vi "Check LVDT's Position.vi"(6 "lvdt display in":T1[](array[typedef]) {"value" format="%.2f"}, 8 "System Error In":errorcluster, 9 "check lvdt x?":bool, 10 "input cluster":T2={"Application Status"="", "Switch Output Array"=[], "Switch Value Configuration"=[], "NVH Configuration"={"NVH Station?"=FALSE, "nvh app instance path"="", "NVH_ErrorMessages sv url"="", "NVH_Inputs sv url"="", "NVH_MotionNumber sv url"="", "NVH_Outputs sv url"="", "NVH_PartNumber sv url"="", "NVH_PartNumber_Echo sv url"="", "NVH_SerialNumber sv url"="", "NVH_AmbientTempF sv url"=""}, "rs232 port map"={"PMAC"="", "PS Port"="", "LVDT Unit"="", "RS232"=""}, "ethernet address map"={"LVDT 1 Unit"="172.17.53.143", "LVDT Unit 1 port"=0}, "paths"={"Base Path"=path "", "system error log path"=path "", "Error Table Path"=path "C/Labview Code/System/Error Table", "Store errors log path"=path "C/Labview Code/System/Error Table", "data bytes log path"=path "C/Labview Code/System/Error Table", "network path"=path "C/Labview Code/System/Error Table"}, "Station Index"=0, "Store Data"={"Motion Data Array"=[], "Error Table"=[], "Sun Shade Close Force Limits"={"Overall Min"=0.0, "Overall Max"=0.0, "Avg Min"=0.0, "Avg Max"=0.0, "Truncation Start"=0.0, "Truncation End"=0.0, "Variance"=0.0, "Check Noise"=FALSE}, "Sun Shade Open Force Limits"={"Overall Min"=0.0, "Overall Max"=0.0, "Avg Min"=0.0, "Avg Max"=0.0, "Truncation Start"=0.0, "Truncation End"=0.0, "Variance"=0.0, "Check Noise"=FALSE}, "Sunshade Open Data"=[], "Sunshade Close Data"=[], "Module Info"={"Serial Number"="", "Pallet Number"="", "Sunshade Color"="", "Inalfa Part Number"="", "Customer Number"=""}, "Sunsahde Close Raw Data"=[], "Sunshade Open Raw Data"=[], "Software Version"=[], "Constant Version"=[], "Hardware Version"=[], "Inalfa Part Number ECU"=[], "LVDT Data"=[], "Communication Line 1"=[], "Communication Line 2"=[], "Anti Pinch Force"=[], "Cycle Time"="", "Anti Pinch Vent Force"=[], "iGPS LVDT Data"=[], "data bytes log"=""}, "D in map"={"Abort Test"=enum."Dev2/port2/line6", "Start Test"=enum."Dev2/port2/line6"}, "DO Task"="", "ctl refs"={"Start Test"=refnum, "Abort Test"=refnum, "Manual Control"=refnum, "Route to Repair"=refnum, "Waveform Graph"=refnum, "Motion Data"=refnum, "all station status"=refnum, "Individual Station Status"=refnum, "exit program"=refnum, "Sunshade Servo Data Open"=refnum, "Sunshade Servo Data Close"=refnum, "Red-Rabbit Mode"=refnum, "Direct Manual Ctrl"=refnum}, "misc station config"={"Station Name"="", "is AT station?"=FALSE, "is audit station?"=FALSE, "power supply type"=enum."GENser", "use alt China TP2 LVDT Logic Seq"=FALSE, "hmi operator abort timeout"=0, "dump all analog values even if pass"=FALSE, "debug log pre-filter ap stream bytes"=FALSE, "use separate lvdt x and z extend tags"=FALSE, "is print"=FALSE}, "ethernet tcp refs"={"LVDT Unit"=refnum}, "Sunshade Barcode Scan"={"Sunshade Number 2"="", "Sunshade Number 1"="", "Keyence tuning bank idx"=0}, "AP Test Data"={"Raw Sunshade AP Data"="", "Raw Glass AP Data"="", "PMAC Read Counter"=0.0, "Database AP Data"=[]}, "Motion Status"={"hmi operator abort start time"=0, "Current Data Index"=0, "Analog Data"=[], "Motor Position Hex"=0, "Messages Index"=0, "Last Bytes"=[], "Current Hall Position"=0, "Motion Stop Timer"=0, "Position Test"=enum."Not Tested", "Noise Test"=enum."Not Tested", "motion stop check initialized"=FALSE, "remote sense enabled"=FALSE, "Motion"=enum."Glass Teach"}, "LVDT Status"={"LVDT's stored config"=[], "lvdt precision"={"truncate instead of rounding"=FALSE, "decimal places"=0}}, "Sequence State"={"Step Description"="", "Cycle Start Time"=0, "Step Data String"="", "Pass?"=FALSE, "Seqence"=[], "Active Step"=0, "Testing?"=FALSE, "Red-Rabbit Mode"=FALSE, "route-to-repair mode"=FALSE, "NVH Status"={"Restart IRQ Counter"=0, "NVH Test Needed?"=FALSE, "NVH Test Running?"=FALSE}, "Present (s)"=0.0, "Hold Mode?"=FALSE, "Hold?"=FALSE, "Rx Invalid?"=FALSE}, "misc status"={"delay start time (ticks)"=0, "In Vehicle Mode?"=FALSE, "Diag Mode?"=FALSE, "Serial Port Configured?"=FALSE, "PS Voltage"=0.0, "Diag Serial Port"="", "Part Setup"={"Communication Type"=enum."None", "Send Messages to"=enum."Glass", "RAP Signal"=enum."High", "Motor Type"=enum."Smart Motor", "NVH Part Number"=0, "Turn Off Timer"=0, "Part Type"=""}, "Part History Number"="", "Plant Number"=0, "AP Data Type"=enum."91/61", "Real Rollo?"=FALSE}, "NVH Operator?"=FALSE, "NVH Pass?"=FALSE, "Operator Pass?"=FALSE, "Operator Action?"=FALSE, "Noise Source"=0, "USBHandle"=0, "PeakInfo"="", "PeakNumber"=0, "NVH Motion Steps"=[], "Second Check?"=FALSE, "Decibel data"=[], "Direct Control Info"={"EnableStopOnHome"=FALSE, "EnableStopOnPos"=FALSE, "TeachEvent"=FALSE, "open offset"=0, "close offset"=0, "Derect control"=FALSE, "set position"=[], "teach pass "=FALSE, "Drift offsets"=[], "Hall Positions"=[]}, "manual control(direct)"=FALSE, "LIN INFO"={"Toolkit Type"=enum."Inalfa LIN", "NAD"=36, "Inalfa LIN"={"Master Frame(3C)"="", "Slave Frame(3D)"="NIXNET_exampleLDF", "Request Schedule"="NIXNET_exampleLDF", "Response Schedule"="CEMLIN3DiagResponseSchedule\nSPA3414_ConfigurationsCMAGeely_CEMCALYPSOSDB34XX0Cfg_LIN3_190709_", "Frame Write SCU"="", "Frame Read SCU"="", "LIN Name"=""}, "ADCS LIN"={"Port"="MasterReq\nSPA3414_ConfigurationsCMAGeely_CEMCALYPSOSDB34XX0Cfg_LIN3_190709_", "HW select"=0, "XNET Cluster"="SlaveResp\nSPA3414_ConfigurationsCMAGeely_CEMCALYPSOSDB34XX0Cfg_LIN3_190709_", "ByteCmd Path"=path "C/Labview Code/System/ByteCmdConfig.txt"}, "TS LIN"={"ref info"=refnum, "LIN Channel"=0, "ByteCmd Path"=path "C/Labview Code/System/ByteCmdConfig.txt"}}, "Config Info"=variant} {"LIN INFO"."NAD" format="%.0x"; "LIN INFO"."ADCS LIN"."HW select" items=["NI-XNET", "NI-CAN"]; "LVDT Status"."LVDT's stored config"."Lower Limit" format="%.2f"; "LVDT Status"."LVDT's stored config"."Upper Limit" format="%.2f"; "Store Data"."Sun Shade Open Force Limits"."Variance" format="%.2g"; "Store Data"."Sun Shade Open Force Limits"."Truncation End" format="%.2g"; "Store Data"."Sun Shade Open Force Limits"."Truncation Start" format="%.2g"; "Store Data"."Sun Shade Open Force Limits"."Avg Max" format="%.2g"; "Store Data"."Sun Shade Open Force Limits"."Avg Min" format="%.2g"; "Store Data"."Sun Shade Open Force Limits"."Overall Max" format="%.2g"; "Store Data"."Sun Shade Open Force Limits"."Overall Min" format="%.2g"; "Store Data"."Sun Shade Close Force Limits"."Variance" format="%.2g"; "Store Data"."Sun Shade Close Force Limits"."Truncation End" format="%.2g"; "Store Data"."Sun Shade Close Force Limits"."Truncation Start" format="%.2g"; "Store Data"."Sun Shade Close Force Limits"."Avg Max" format="%.2g"; "Store Data"."Sun Shade Close Force Limits"."Avg Min" format="%.2g"; "Store Data"."Sun Shade Close Force Limits"."Overall Max" format="%.2g"; "Store Data"."Sun Shade Close Force Limits"."Overall Min" format="%.2g"}, 11 "Database LVDT's Data In":sgl[](array[numeric])) -> (0 "System Error Out":errorcluster, 1 "Error String Number":u16[](array[numeric]), 2 "Error String Array":string[](array[string]), 3 "Database LVDT's Data Out":sgl[](array[numeric]), 4 "lvdt display out":T1[](array[typedef]) {"value" format="%.2f"}, 5 "Pass?":bool)   [LabVIEW 2018]
uses:
  type defs/EOL LVDT's Check Controller.ctl
  02.Type Def's/lvdt name val pair.ctl
  <vilib>/Platform/dataskt.llb/DataSocket Reference Type.ctl
  type defs/plc path and tag.ctl
  02.Type Def's/station plc write boolean tags.ctl
  02.Type Def's/station plc read boolean tags.ctl
  type defs/EOL Global Digital Input Control.ctl
  02.Type Def's/station DI map.ctl
  lvdt precision.ctl
  02.Type Def's/All Communication Types.ctl
  type defs/Communication with Motors.ctl
  type defs/RAP Signal Control.ctl
  type defs/EOL Motor Type.ctl
  type defs/EOL Part Setup.ctl
  type defs/17x AP Data Type.ctl
  02.Type Def's/All Motions.ctl
  02.Type Def's/EOL Switch Max Min Check Cluster.ctl
  02.Type Def's/EOL Switch Value Configuration Cluster.ctl
  02.Type Def's/All Switch Configuration Cluster.ctl
  type defs/17x Sunshade Limts Seq.ctl
  02.Type Def's/Pass Fail Control.ctl
  02.Type Def's/EOL Module Info Control.ctl
  type defs/17x Audit Motion Data Seq Control.ctl
  02.Type Def's/EOL Motion Database Table.ctl
  sequence/type defs/Sequence Info.ctl
  02.Type Def's/station nvh config.ctl
  02.Type Def's/station rs232 port map.ctl
  02.Type Def's/station ethernet address map.ctl
  02.Type Def's/station paths.ctl
  02.Type Def's/EOL Save Module Test Data Control.ctl
  02.Type Def's/Screen Motion Data.ctl
  02.Type Def's/station motion data indicator.ctl
  02.Type Def's/station hmi.ctl
  02.Type Def's/individual station status.ctl
  02.Type Def's/control refs.ctl
  Lambda Power/power supply types.ctl
  02.Type Def's/main state cluster.ctl
  02.Type Def's/sequence state.ctl
  03.Inalfa LIN/LIN Device.ctl
  <vilib>/CMC.AME/Inalfa ADCS/Ctl'Def/ADCS_LIN info.ctl
  02.Type Def's/station LIN config.ctl
  02.Type Def's/misc station config.ctl
  06.Test Loop/Sub'VIs/Type Def's/Config Info.ctl
  C:/Program Files (x86)/National Instruments/LabVIEW 2018/vi.lib/CMC.AME/Inalfa TS LIN/TOSUN/TSMaster/bin/Interop.TSMasterAPI.dll
  Program Files (x86)/National Instruments/LabVIEW 2018/vi.lib/CMC.AME/Inalfa TS LIN/TOSUN/TSMaster/bin/Interop.TSMasterAPI.dll
panel:
  # "Sunroof Barcode"
  # "Pallet Number"
  # "Part Type"
  # "Application Status"
  # "Current Step"
  # "Cycle Time"
  # "Pass / Fail"
  # "Shade Close"
  # "Actual Data"
  # "Limits"
  # "Avg Current"
  # "Run Time"
  # "Speed"
  # "Noise Test"
  # "Position"
  # "Shade Open"
  # "Actual Data"
  # "Limits"
  # "Avg Current"
  # "Run Time"
  # "Speed"
  # "Noise Test"
  # "Position"
  # "Vent Close"
  # "Actual Data"
  # "Limits"
  # "Avg Current"
  # "Run Time"
  # "Speed"
  # "Noise Test"
  # "Position"
  # "Vent Open"
  # "Actual Data"
  # "Limits"
  # "Avg Current"
  # "Run Time"
  # "Speed"
  # "Noise Test"
  # "Position"
  # "Slide Close"
  # "Actual Data"
  # "Limits"
  # "Avg Current"
  # "Run Time"
  # "Speed"
  # "Noise Test"
  # "Position"
  # "Slide Open"
  # "Actual Data"
  # "Limits"
  # "Avg Current"
  # "Run Time"
  # "Speed"
  # "Noise Test"
  # "Position"
  # "Min"
  # "N"
  # "Min"
  # "Start"
  # "N"
  # "Max"
  # "N"
  # "Max"
  # "N"
  # "End"
  # "Min"
  # "N"
  # "Min"
  # "Start"
  # "N"
  # "Max"
  # "N"
  # "Max"
  # "N"
  # "End"
  # "Min"
  # "Max"
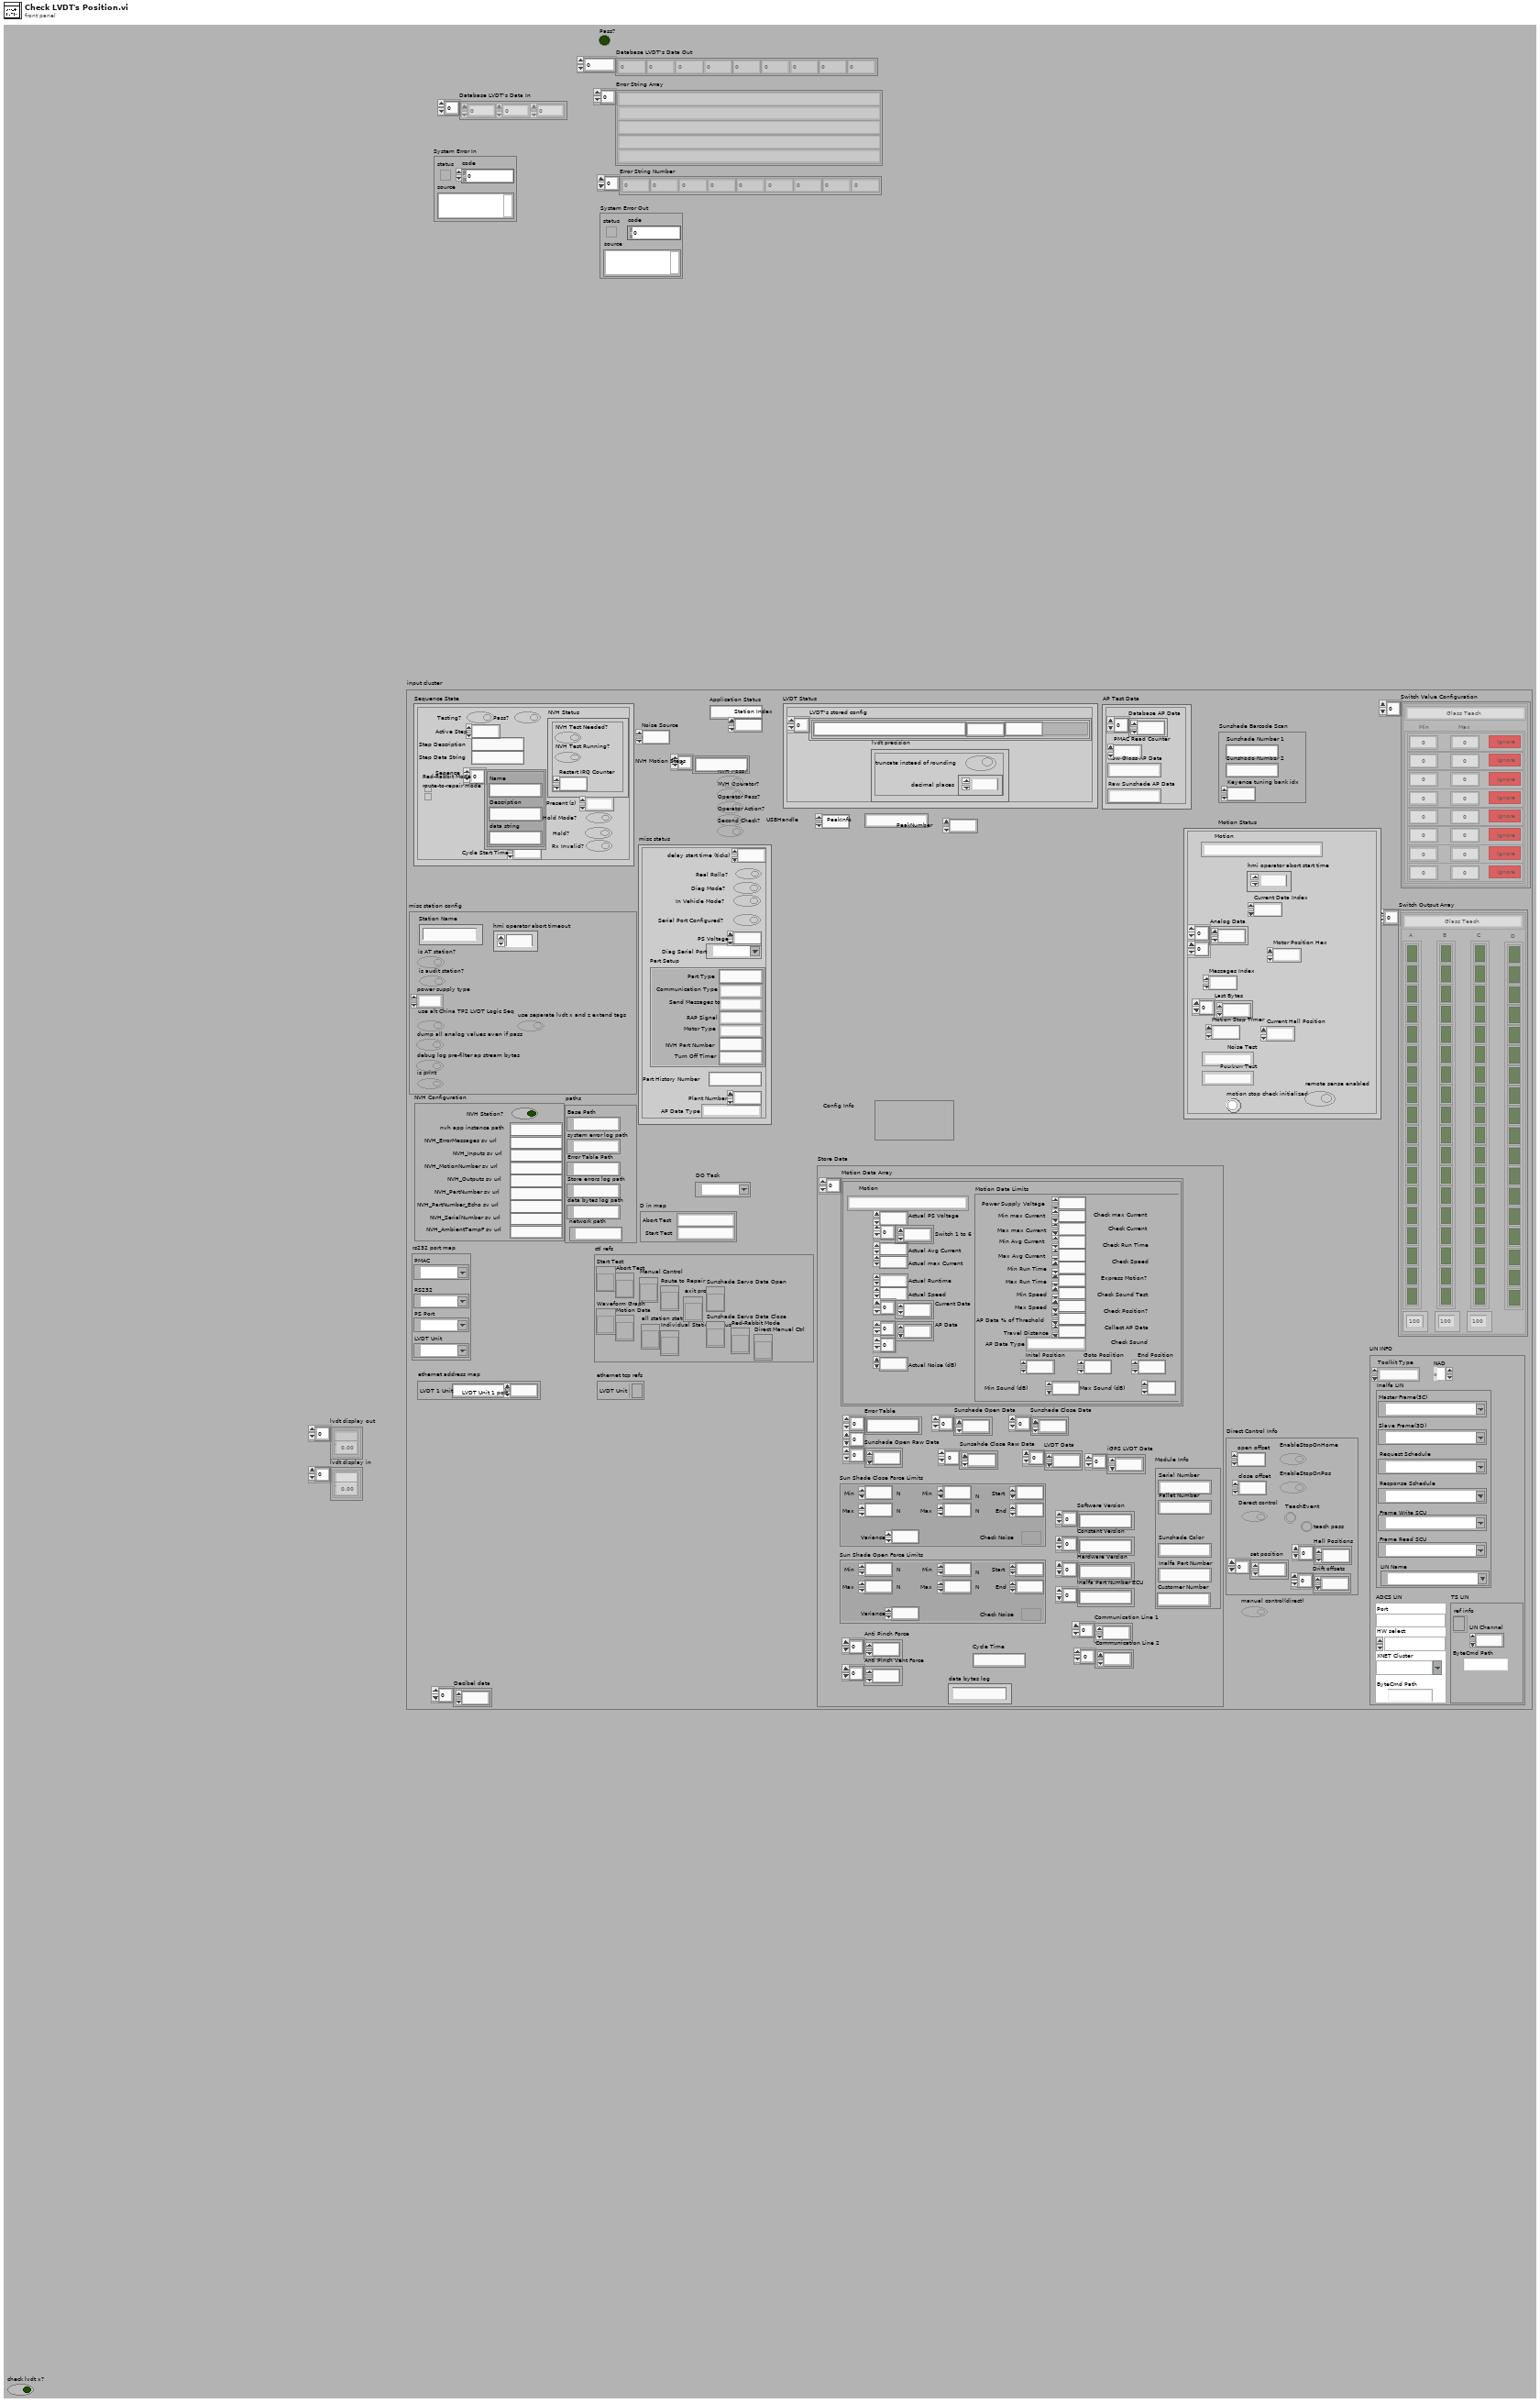
[diagram p1: front panel]
types:
  T1 = typedef "lvdt name val pair.ctl" = cluster{"lvdt name":string, "value":dbl}
  T2 = typedef "main state cluster.ctl" = cluster{"Application Status":string, "Switch Output Array":T3[], "Switch Value Configuration":T5[], "NVH Configuration":T7, "rs232 port map":T8, "ethernet address map":T9, "paths":T10, "Station Index":i32, "Store Data":T11, "D in map":T17, "DO Task":refnum<k21>, "ctl refs":T19, "misc station config":T20, "ethernet tcp refs":cluster{"LVDT Unit":refnum<k5>}, "Sunshade Barcode Scan":cluster{"Sunshade Number 2":string, "Sunshade Number 1":string, "Keyence tuning bank idx":i32}, "AP Test Data":cluster{"Raw Sunshade AP Data":string, "Raw Glass AP Data":string, "PMAC Read Counter":dbl, "Database AP Data":dbl[]}, "Motion Status":cluster{"hmi operator abort start time":u32, "Current Data Index":i32, "Analog Data":sgl[][], "Motor Position Hex":u16, "Messages Index":u16, "Last Bytes":u8[], "Current Hall Position":i16, "Motion Stop Timer":u32, "Position Test":T22, "Noise Test":T22, "motion stop check initialized":bool, "remote sense enabled":bool, "Motion":T4}, "LVDT Status":cluster{"LVDT's stored config":T23[], "lvdt precision":T24}, "Sequence State":T25, "misc status":cluster{"delay start time (ticks)":u32, "In Vehicle Mode?":bool, "Diag Mode?":bool, "Serial Port Configured?":bool, "PS Voltage":dbl, "Diag Serial Port":refnum<visa-resource-name>, "Part Setup":T27, "Part History Number":string, "Plant Number":u8, "AP Data Type":T14, "Real Rollo?":bool}, "NVH Operator?":bool, "NVH Pass?":bool, "Operator Pass?":bool, "Operator Action?":bool, "Noise Source":u32, "USBHandle":i32, "PeakInfo":string, "PeakNumber":i32, "NVH Motion Steps":string[], "Second Check?":bool, "Decibel data":dbl[], "Direct Control Info":cluster{"EnableStopOnHome":bool, "EnableStopOnPos":bool, "TeachEvent":bool, "open offset":i32, "close offset":i32, "Derect control":bool, "set position":i32[], "teach pass ":bool, "Drift offsets":i32[], "Hall Positions":i32[]}, "manual control(direct)":bool, "LIN INFO":T32, "Config Info":T35}
  T3 = typedef "All Switch Configuration Cluster.ctl" = cluster{"All Motions":T4, "A":bool[], "B":bool[], "C":bool[], "D":bool[], "A activation time (ms)":u32, "B activation time (ms)":u32, "C activation time (ms)":u32}
  T4 = typedef "All Motions.ctl" = enum16{"Glass Teach", "Glass Slide Open", "Glass Slide Close", "Glass Vent Open", "Glass Vent Close", "Sunshade Teach", "Sunshade Open", "Sunshade Close", "Idle", "Sunshade Open 2", "Sunshade Close 2", "Glass Slide Open Sunshade Open", "Glass Slide Open Sunshade Close", "Glass Slide Close Sunshade Open", "Glass Slide Close Sunshade Close", "Glass Vent Open Sunshade Open", "Glass Vent Open Sunshade Close", "Glass Vent Close Sunshade Open", "Glass Vent Close Sunshade Close", "Express Glass Slide Open", "Express Glass Slide Close", "Express Glass Vent Open", "Express Glass Vent Close", "Express Sunshade Open", "Express Sunshade Close", "Express Sunshade Open 2", "Express Sunshade Close 2", "Express Glass Slide Open Sunshade Open", "Express Glass Slide Open Sunshade Close", "Express Glass Slide Close Sunshade Open", "Express Glass Slide Close Sunshade Close", "Express Glass Vent Open Sunshade Open", "Express Glass Vent Open Sunshade Close", "Express Glass Vent Close Sunshade Open", "Express Glass Vent Close Sunshade Close", "Goto Position Glass", "Goto Position Sunshade", "Sunshade Teach 2"}
  T5 = typedef "EOL Switch Value Configuration Cluster.ctl" = cluster{"All Motions":T4, "Array":T6[]}
  T6 = typedef "EOL Switch Max Min Check Cluster.ctl" = cluster{"Min":dbl, "Max":dbl, "Check?":bool}
  T7 = typedef "station nvh config.ctl" = cluster{"NVH Station?":bool, "nvh app instance path":string, "NVH_ErrorMessages sv url":string, "NVH_Inputs sv url":string, "NVH_MotionNumber sv url":string, "NVH_Outputs sv url":string, "NVH_PartNumber sv url":string, "NVH_PartNumber_Echo sv url":string, "NVH_SerialNumber sv url":string, "NVH_AmbientTempF sv url":string}
  T8 = typedef "station rs232 port map.ctl" = cluster{"PMAC":refnum<visa-resource-name>, "PS Port":refnum<visa-resource-name>, "LVDT Unit":refnum<visa-resource-name>, "RS232":refnum<visa-resource-name>}
  T9 = typedef "station ethernet address map.ctl" = cluster{"LVDT 1 Unit":string, "LVDT Unit 1 port":u16}
  T10 = typedef "station paths.ctl" = cluster{"Base Path":path, "system error log path":path, "Error Table Path":path, "Store errors log path":path, "data bytes log path":path, "network path":path}
  T11 = typedef "EOL Save Module Test Data Control.ctl" = cluster{"Motion Data Array":T12[], "Error Table":string[][], "Sun Shade Close Force Limits":T15, "Sun Shade Open Force Limits":T15, "Sunshade Open Data":sgl[], "Sunshade Close Data":sgl[], "Module Info":T16, "Sunsahde Close Raw Data":sgl[], "Sunshade Open Raw Data":sgl[], "Software Version":string[], "Constant Version":string[], "Hardware Version":string[], "Inalfa Part Number ECU":string[], "LVDT Data":sgl[], "Communication Line 1":sgl[], "Communication Line 2":sgl[], "Anti Pinch Force":sgl[], "Cycle Time":string, "Anti Pinch Vent Force":sgl[], "iGPS LVDT Data":sgl[], "data bytes log":string}
  T12 = typedef "EOL Motion Database Table.ctl" = cluster{"Motion":T4, "Actual Avg Current":dbl, "Actual Runtime":dbl, "Actual Speed":dbl, "Current Data":sgl[], "Motion Data Limits":T13, "Switch 1 to 6":dbl[], "Actual PS Voltage":dbl, "AP Data":i16[][], "Actual max Current":dbl, "Actual Noise (dB)":dbl}
  T13 = typedef "17x Audit Motion Data Seq Control.ctl" = cluster{"Power Supply Voltage":dbl, "Min Avg Current":dbl, "Max Avg Current":dbl, "Min Run Time":dbl, "Max Run Time":dbl, "Min Speed":dbl, "Max Speed":dbl, "AP Data % of Threshold":dbl, "Travel Distance":dbl, "AP Data Type":T14, "Check Current":bool, "Check Run Time":bool, "Check Speed":bool, "Express Motion?":bool, "Check Sound Test":bool, "Check Position?":bool, "Collect AP Data":bool, "Inital Position":u16, "End Position":u16, "Goto Posiition":u16, "Max max Current":dbl, "Min max Current":dbl, "Check max Current":bool, "Check Sound":bool, "Min Sound (dB)":dbl, "Max Sound (dB)":dbl}
  T14 = typedef "17x AP Data Type.ctl" = enum16{"91/61", "92/62", "93/63", "67", "68", "6F", "71", "91 Msg", "92 Msg", "93 Msg", "94 Msg", "HiRain 91", "HiRain 92 Speed", "HiRain 92 HS", "HiRain 92", "HiRain 93", "SnT"}
  T15 = typedef "17x Sunshade Limts Seq.ctl" = cluster{"Overall Min":dbl, "Overall Max":dbl, "Avg Min":dbl, "Avg Max":dbl, "Truncation Start":dbl, "Truncation End":dbl, "Variance":dbl, "Check Noise":bool}
  T16 = typedef "EOL Module Info Control.ctl" = cluster{"Serial Number":string, "Pallet Number":string, "Sunshade Color":string, "Inalfa Part Number":string, "Customer Number":string}
  T17 = typedef "station DI map.ctl" = cluster{"Abort Test":T18, "Start Test":T18}
  T18 = typedef "EOL Global Digital Input Control.ctl" = enum16{"Dev2/port0/line0", "Dev2/port0/line1", "Dev2/port0/line2", "Dev2/port0/line3", "Dev2/port0/line4", "Dev2/port0/line5", "Dev2/port0/line6", "Dev2/port0/line7", "Dev2/port1/line0", "Dev2/port1/line1", "Dev2/port1/line2", "Dev2/port1/line3", "Dev2/port1/line4", "Dev2/port1/line5", "Dev2/port1/line6", "Dev2/port1/line7", "Dev2/port2/line0", "Dev2/port2/line1", "Dev2/port2/line2", "Dev2/port2/line3", "Dev2/port2/line4", "Dev2/port2/line5", "Dev2/port2/line6", "Dev2/port2/line7", "Prerun Start Test", "Prerun Abort Test", "Audit Start Test", "Audit Abort Test", "Dev2/port3/line4", "Dev2/port3/line5", "Breakin Start Test", "Breakin Abort Test", "Not Implemented"}
  T19 = typedef "control refs.ctl" = cluster{"Start Test":refnum<vi>, "Abort Test":refnum<vi>, "Manual Control":refnum<vi>, "Route to Repair":refnum<vi>, "Waveform Graph":refnum<vi>, "Motion Data":refnum<vi>, "all station status":refnum<vi>, "Individual Station Status":refnum<vi>, "exit program":refnum<vi>, "Sunshade Servo Data Open":refnum<vi>, "Sunshade Servo Data Close":refnum<vi>, "Red-Rabbit Mode":refnum<vi>, "Direct Manual Ctrl":refnum<vi>}
  T20 = typedef "misc station config.ctl" = cluster{"Station Name":string, "is AT station?":bool, "is audit station?":bool, "power supply type":T21, "use alt China TP2 LVDT Logic Seq":bool, "hmi operator abort timeout":u32, "dump all analog values even if pass":bool, "debug log pre-filter ap stream bytes":bool, "use separate lvdt x and z extend tags":bool, "is print":bool}
  T21 = typedef "power supply types.ctl" = enum16{"GENser", "ZUPser", "GENeth", "Manual", "ITECH"}
  T22 = typedef "Pass Fail Control.ctl" = enum16{"Not Tested", "Pass", "Fail"}
  T23 = typedef "EOL LVDT's Check Controller.ctl" = cluster{"Upper Limit":dbl, "Lower Limit":dbl, "LVDT Name":string, "Check":bool}
  T24 = typedef "lvdt precision.ctl" = cluster{"truncate instead of rounding":bool, "decimal places":u8}
  T25 = typedef "sequence state.ctl" = cluster{"Step Description":string, "Cycle Start Time":u32, "Step Data String":string, "Pass?":bool, "Seqence":T26[], "Active Step":u8, "Testing?":bool, "Red-Rabbit Mode":bool, "route-to-repair mode":bool, "NVH Status":cluster{"Restart IRQ Counter":u8, "NVH Test Needed?":bool, "NVH Test Running?":bool}, "Present (s)":dbl, "Hold Mode?":bool, "Hold?":bool, "Rx Invalid?":bool}
  T26 = typedef "Sequence Info.ctl" = cluster{"Name":string, "Description":string, "data string":string}
  T27 = typedef "EOL Part Setup.ctl" = cluster{"Communication Type":T28, "Send Messages to":T29, "RAP Signal":T30, "Motor Type":T31, "NVH Part Number":u16, "Turn Off Timer":u16, "Part Type":string}
  T28 = typedef "All Communication Types.ctl" = enum16{"None", "CAN", "RS 232", "RS 232 LIN", "GM LIN", "SnT LIN", "K Line", "Robel CAN", "P42M-Continental", "Inalfa SCU LIN", "Spare 3"}
  T29 = typedef "Communication with Motors.ctl" = enum16{"Glass", "Rollo", "Both"}
  T30 = typedef "RAP Signal Control.ctl" = enum16{"High", "Low", "None"}
  T31 = typedef "EOL Motor Type.ctl" = enum16{"Smart Motor", "Sensor Motor"}
  T32 = typedef "station LIN config.ctl" = cluster{"Toolkit Type":enum16{"Inalfa LIN", "ADCS LIN", "TS LIN"}, "NAD":u8, "Inalfa LIN":T33, "ADCS LIN":T34, "TS LIN":cluster{"ref info":refnum<k24>, "LIN Channel":i32, "ByteCmd Path":path}}
  T33 = typedef "LIN Device.ctl" = cluster{"Master Frame(3C)":refnum<k21>, "Slave Frame(3D)":refnum<k21>, "Request Schedule":refnum<k21>, "Response Schedule":refnum<k21>, "Frame Write SCU":refnum<k21>, "Frame Read SCU":refnum<k21>, "LIN Name":refnum<k21>}
  T34 = typedef "ADCS_LIN info.ctl" = cluster{"Port":string, "HW select":u16, "XNET Cluster":string, "ByteCmd Path":path}
  T35 = typedef "Config Info.ctl" = variant
  T36 = typedef "station plc write boolean tags.ctl" = cluster{"AT set glass wand lower":T37, "AT set sunshade wand lower":T37, "AT set wand home pos":T37, "Test Complete Pass":T37, "Test Complete Fail":T37, "Test Started":T37, "Retract LVDT's":T37, "Extend LVDT's":T37, "ss servo open":T37, "ss servo close":T37, "control slide start":T37, "control slide stop":T37, "AT VentPMACHome":T37, "AT VentPMACExtended":T37, "Good Frame Barcode":T37, "Bad Frame Barcode":T37, "Extend Z LVDTS":T37, "NVH SunRoof Moving":T37, "NVH SunRoof Stop":T37, "NVH Pass":T37, "NVH Fail":T37, "NVH Operator Express Glass Opened":T37, "NVH Operator Express Glass Closed":T37, "NVH Operator Express Rollo Opened01":T37, "NVH Operator Express Rollo Closed01":T37, "NVH Operator Express Rollo Opened02":T37, "NVH Operator Pass":T37, "NVH Operator Fail":T37, "NVH Operator Check":T37, "NVH Operator Vent Open Noise":T37, "NVH Operator Vent Close Noise":T37, "NVH Operator Sunshade Open Noise":T37, "NVH Operator Sunshade Close Noise":T37, "NVH Operator Glass Open Noise":T37, "NVH Operator Glass Close Noise":T37, "NVH Operator Finish":T37, "AT set sunshade 02 wand up":T37, "AT set wand 02 home pos":T37, "Barcode01 OK":T37, "Barcode02 OK":T37, "AT set to Vent ATS Test Pos":T37, "AT set to Vent ATS Home Pos":T37, "Move LVDT Adjust Station":T37}
  T37 = typedef "plc path and tag.ctl" = cluster{"Tag Name":string, "Network Path":string, "use opc":bool, "DataSocket Reference":T38}
  T38 = typedef "DataSocket Reference Type.ctl" = cluster{"CWDSLib._DCWDataSocket":refnum<k7>, "CWDSLib._DCWData":refnum<k7>, "OnDataUpdated":u32, "OnStatusUpdated":u32}
  T39 = typedef "station plc read boolean tags.ctl" = cluster{"AT glass position":T37, "AT shade position":T37, "AT in glass wand lower pos":T37, "AT in sunshad wand lower pos":T37, "AT in wand home pos":T37, "LVDT's Extended":T37, "motor foam present LH":T37, "motor foam present RH":T37, "audit gap hider present LH":T37, "audit gap hider present RH":T37, "FB light block present":T37, "bolt check 1":T37, "bolt check 2":T37, "bolt check 3":T37, "bolt check 4":T37, "bolt check 5":T37, "bolt check 6":T37, "bolt check 7":T37, "bolt check 8":T37, "bolt check 9":T37, "bolt check 10":T37, "bolt check 11":T37, "bolt check 12":T37, "bolt check 13":T37, "bolt check 14":T37, "bolt check 15":T37, "bolt check 16":T37, "bolt check 17":T37, "bolt check 18":T37, "bolt check 19":T37, "bolt check 20":T37, "bolt check 21":T37, "start":T37, "abort":T37, "LVDT's Retracted":T37, "manual barcode print":T37, "ss servo at open":T37, "ss servo at close":T37, "ss servo opening":T37, "ss servo closing":T37, "control slide at home":T37, "control slide left good":T37, "control slide left over stroke":T37, "control slide right good":T37, "control slide right over stroke":T37, "wind deflector high speed pos":T37, "wind deflector low speed pos":T37, "AT VentPMACatHome":T37, "AT VentPMACisExtend":T37, "SS Barcode Scanner Bypassed":T37, "Check Frame Barcode":T37, "iGPS Pass 0":T37, "iGPS Pass 1":T37, "iGPS Pass 2":T37, "iGPS Pass 3":T37, "iGPS Pass 4":T37, "iGPS Pass 5":T37, "iGPS Pass 6":T37, "iGPS Pass 7":T37, "iGPS Pass 8":T37, "iGPS Pass 9":T37, "Z LVDTs Extended":T37, "NVH Operator Pass":T37, "NVH Operator Fail":T37, "NVH Operator Express Glass Open":T37, "NVH Operator Express Glass Close":T37, "NVH Operator Express Rollo Open01":T37, "NVH Operator Express Rollo Close01":T37, "NVH Operator Express Rollo Open02":T37, "NVH Operator Express Rollo Close02":T37, "NVH Operator Vent Open Noise":T37, "NVH Operator Vent Close Noise":T37, "NVH Operator Sunshade Open Noise":T37, "NVH Operator Sunshade Close Noise":T37, "NVH Operator Glass Open Noise":T37, "NVH Operator Glass Close Noise":T37, "NVH Operator Finish":T37, "NVH Operator Check":T37, "AT shade 02 position":T37, "AT in sunshad 02 wand up pos":T37, "AT in wand 02 home pos":T37, "windproof position":T37, "NVH Operator Express Glass vent Open":T37, "NVH Operator Express Glass Vent Close":T37, "NVH Operator Re-do":T37, "AT at vent ATS test pos":T37, "AT at vent ATS Home pos":T37, "Start Adjust LVDT":T37, "Finish Adjust LVDT":T37}
  T40 = cluster{"Pass?":bool, "LVDT Unit 1":refnum<visa-resource-name>, "LVDT Data String":string, "LVDT's Data Array":sgl[], "LVDT's Limits":T23[], "Error String Array":string[], "Error String Number":u16[], "System Error In":errorcluster, "Step Data String":string, "PLC bool write Tags":T36, "PLC boolean read Tags":T39, "D in map":T17, "LVDT's stored config":T23[], "lvdt precision":T24, "LVDT Unit 1 ip":string, "use alt China TP2 LVDT Logic Seq":bool, "check lvdt x?":bool, "separate z extend":bool, "misc status":cluster{"delay start time (ticks)":u32, "In Vehicle Mode?":bool, "Diag Mode?":bool, "Serial Port Configured?":bool, "PS Voltage":dbl, "Diag Serial Port":refnum<visa-resource-name>, "Part Setup":T27, "Part History Number":string, "Plant Number":u8, "AP Data Type":T14, "Real Rollo?":bool}}
  T41 = typedef "plc comms params.ctl" = cluster{"PLC boolean read Tags":T42, "PLC bool write Tags":T36, "PLC string read Tags":T43, "PLC string write Tags":T44, "use opc":bool, "PLC/OPC Path":string, "PLC float read Tags":T45}
  T42 = typedef "station plc read boolean tags.ctl" = cluster{"AT glass position":T37, "AT shade position":T37, "AT in glass wand lower pos":T37, "AT in sunshad wand lower pos":T37, "AT in wand home pos":T37, "LVDT's Extended":T37, "bolt check 1":T37, "bolt check 2":T37, "bolt check 3":T37, "bolt check 4":T37, "bolt check 5":T37, "bolt check 6":T37, "bolt check 7":T37, "bolt check 8":T37, "start":T37, "abort":T37, "LVDT's Retracted":T37, "manual barcode print":T37, "ss servo at open":T37, "ss servo at close":T37, "ss servo opening":T37, "ss servo closing":T37, "control slide at home":T37, "control slide left good":T37, "control slide left over stroke":T37, "control slide right good":T37, "control slide right over stroke":T37, "wind deflector high speed pos":T37, "wind deflector low speed pos":T37, "AT VentPMACatHome":T37, "AT VentPMACisExtend":T37, "SS Barcode Scanner Bypassed":T37, "Check Frame Barcode":T37, "Z LVDTs Extended":T37, "NVH Operator Pass":T37, "NVH Operator Fail":T37, "NVH Operator Express Glass Open":T37, "NVH Operator Express Glass Close":T37, "NVH Operator Express Rollo Open01":T37, "NVH Operator Express Rollo Close01":T37, "NVH Operator Express Rollo Open02":T37, "NVH Operator Express Rollo Close02":T37, "NVH Operator Vent Open Noise":T37, "NVH Operator Vent Close Noise":T37, "NVH Operator Sunshade Open Noise":T37, "NVH Operator Sunshade Close Noise":T37, "NVH Operator Glass Open Noise":T37, "NVH Operator Glass Close Noise":T37, "NVH Operator Finish":T37, "NVH Operator Check":T37, "windproof position":T37, "NVH Operator Express Glass vent Open":T37, "NVH Operator Express Glass Vent Close":T37, "NVH Operator Re-do":T37, "AT at vent ATS test pos":T37, "AT at vent ATS Home pos":T37, "Start Adjust LVDT":T37, "Finish Adjust LVDT":T37}
  T43 = typedef "station plc read string tags.ctl" = cluster{"Serial Number":T37, "Pallet Number":T37, "Inalfa Part Number":T37, "Shade Color":T37, "Model Type":T37, "Customer Number":T37, "Part History Number":T37, "Shade 1 Barcode":T37, "Shade 2 Barcode":T37, "Manual Serial Number":T37, "Manual Inalfa Part Number":T37, "Manual Shade Color":T37, "Manual Model Type":T37, "Manual Customer Number":T37, "Manual Part History Number":T37, "iGPS SN 0":T37, "iGPS SN 1":T37, "iGPS SN 2":T37, "iGPS SN 3":T37, "iGPS SN 4":T37, "iGPS SN 5":T37, "iGPS SN 6":T37, "iGPS SN 7":T37, "iGPS SN 8":T37, "iGPS SN 9":T37}
  T44 = typedef "station plc write string tags.ctl" = cluster{"barcode station error":T37, "error message 0":T37, "error message 1":T37, "error message 2":T37, "error message 3":T37, "error message 4":T37, "error message 5":T37, "error message 6":T37, "error message 7":T37, "error message 8":T37, "error message 9":T37}
  T45 = typedef "station plc read float tags.ctl" = cluster{"iGPS float read tags":T46[]}
  T46 = typedef "iGPS float tags.ctl" = cluster{"LVDT measurements":cluster{"value":T37, "UCL":T37, "LCL":T37, "LVDT Name":string}[]}
  T47 = cluster{"delay start time (ticks)":u32, "In Vehicle Mode?":bool, "Diag Mode?":bool, "Serial Port Configured?":bool, "PS Voltage":dbl, "Diag Serial Port":refnum<visa-resource-name>, "Part Setup":T27, "Part History Number":string, "Plant Number":u8, "AP Data Type":T14, "Real Rollo?":bool}
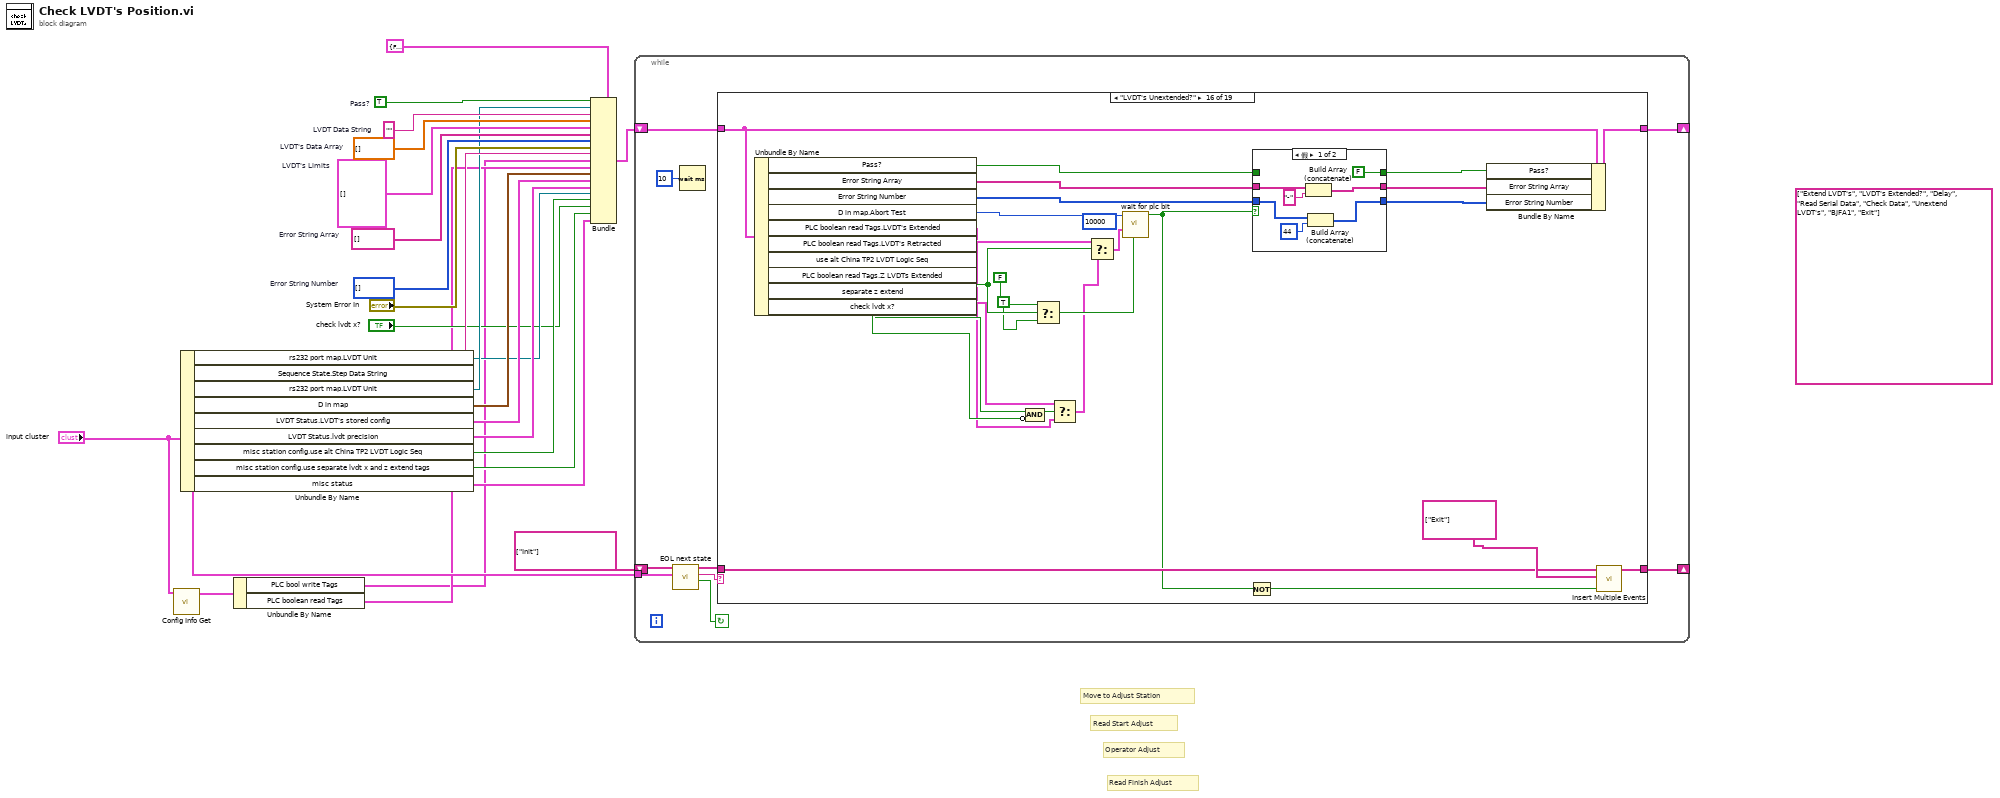
[diagram p0: block diagram]
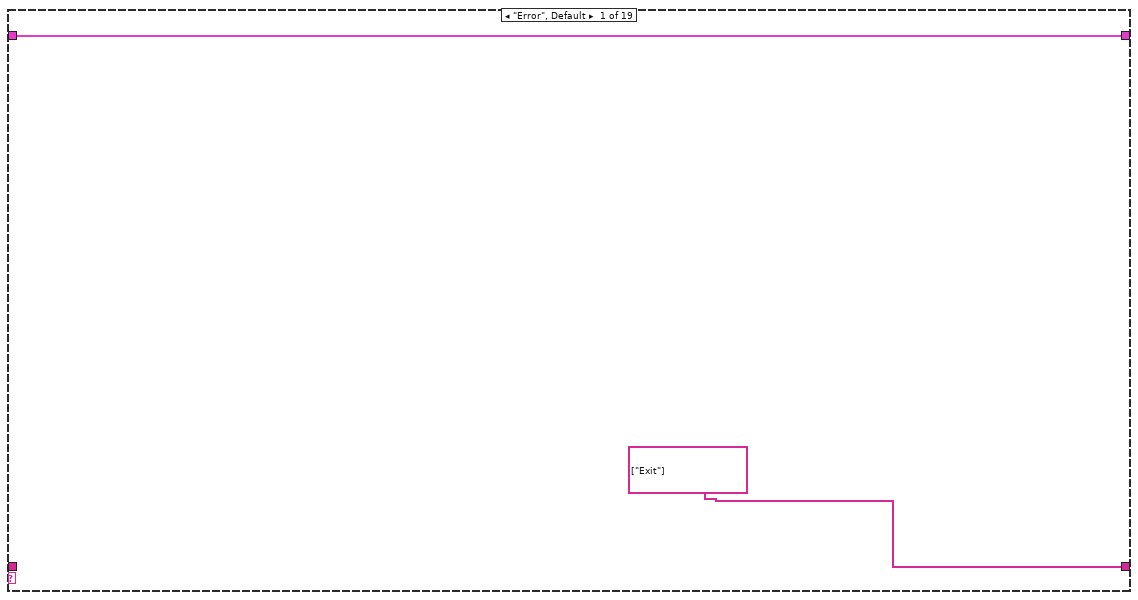
[diagram p2: hidden frame]
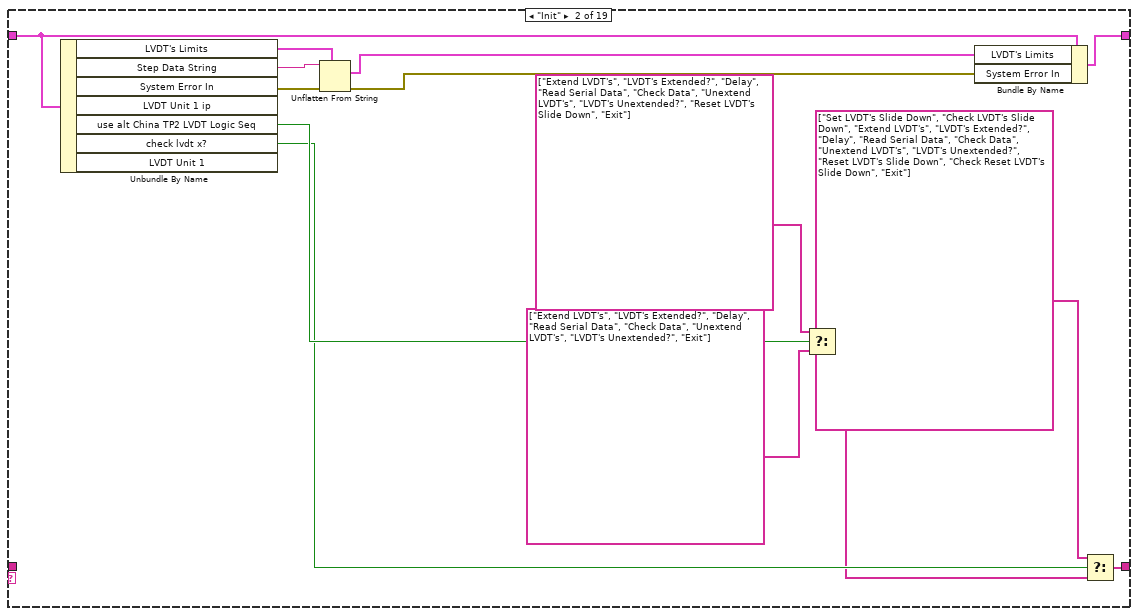
[diagram p3: hidden frame]
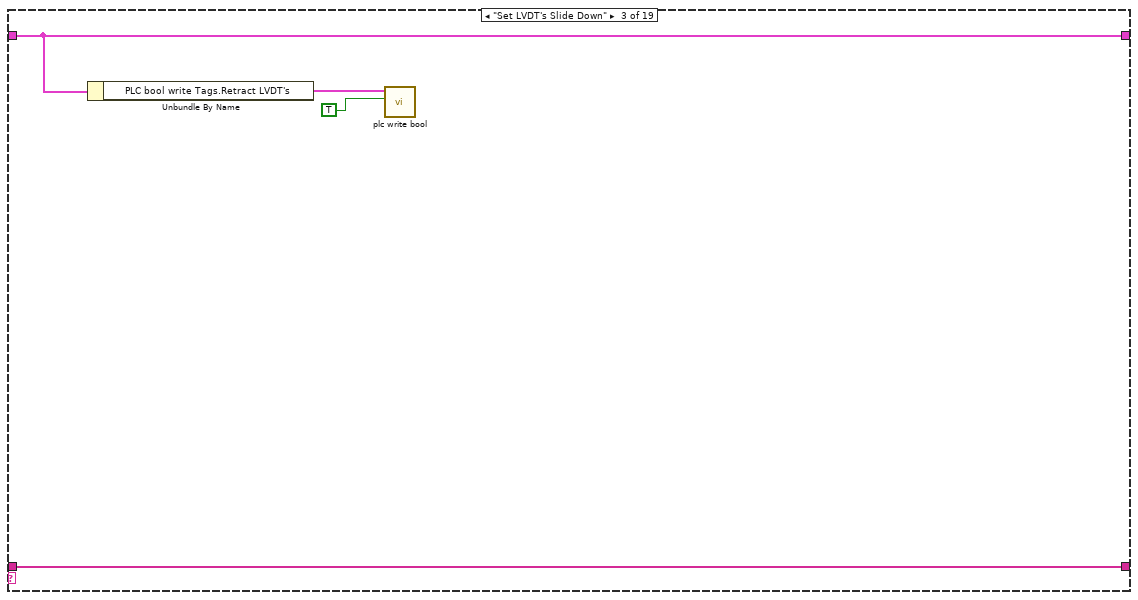
[diagram p4: hidden frame]
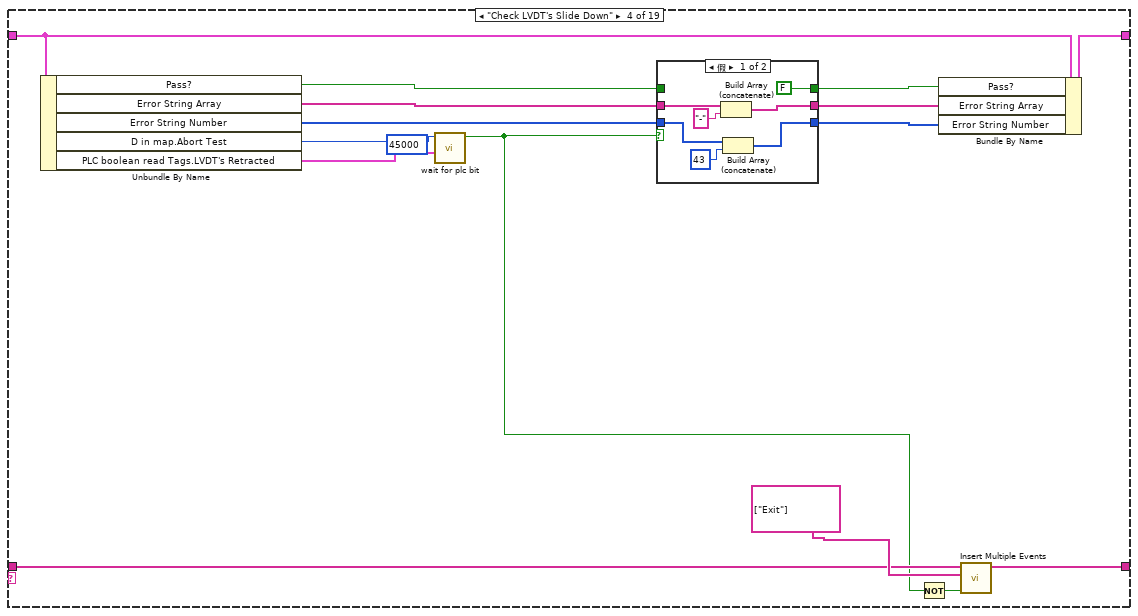
[diagram p5: hidden frame]
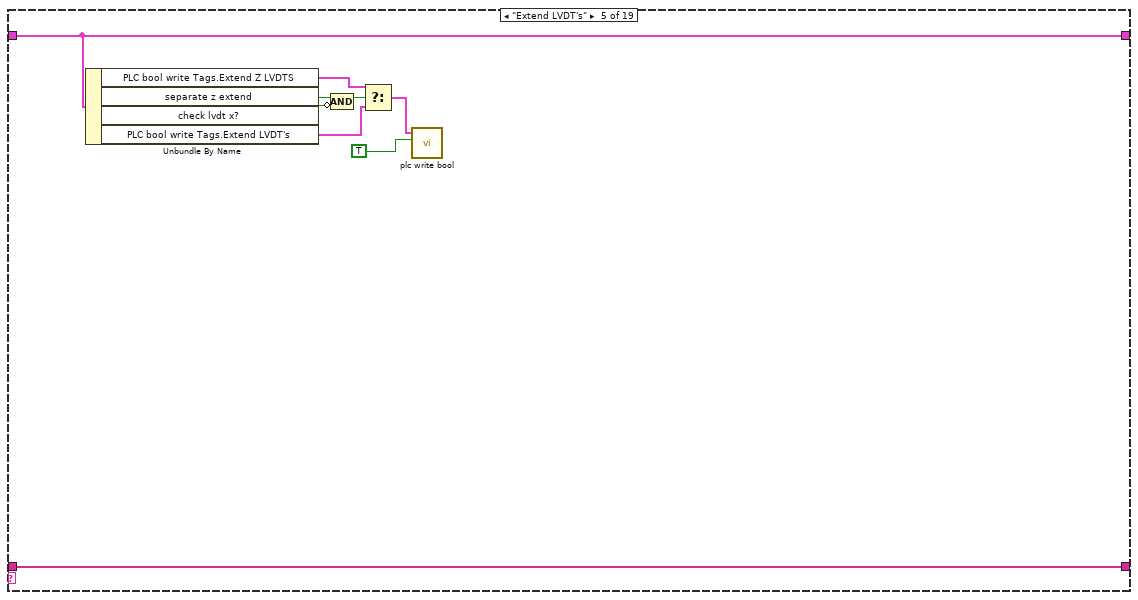
[diagram p7: hidden frame]
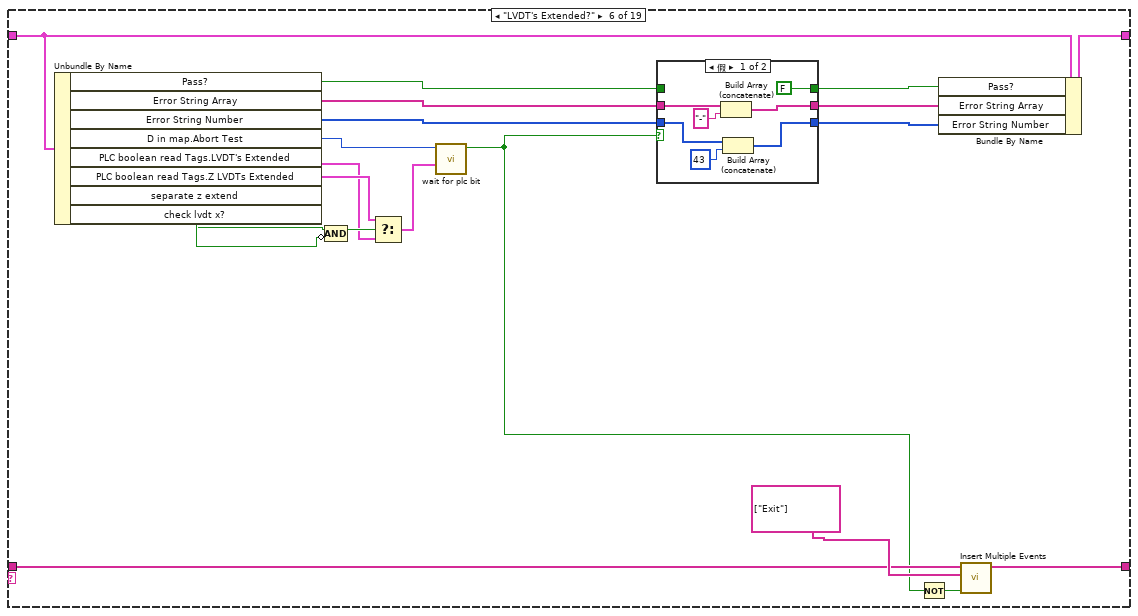
[diagram p8: hidden frame]
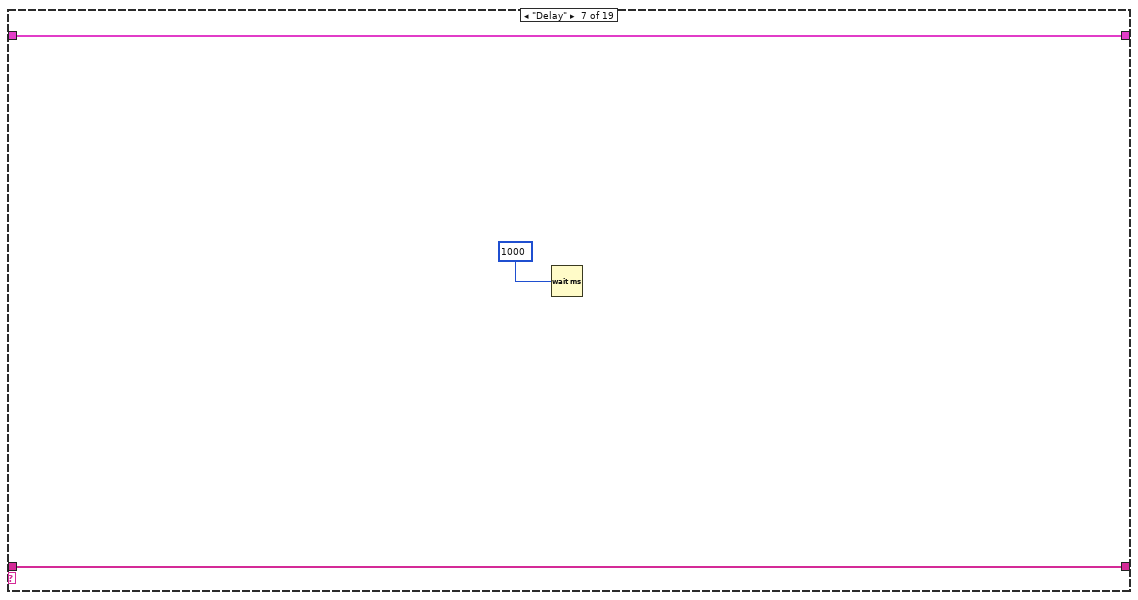
[diagram p10: hidden frame]
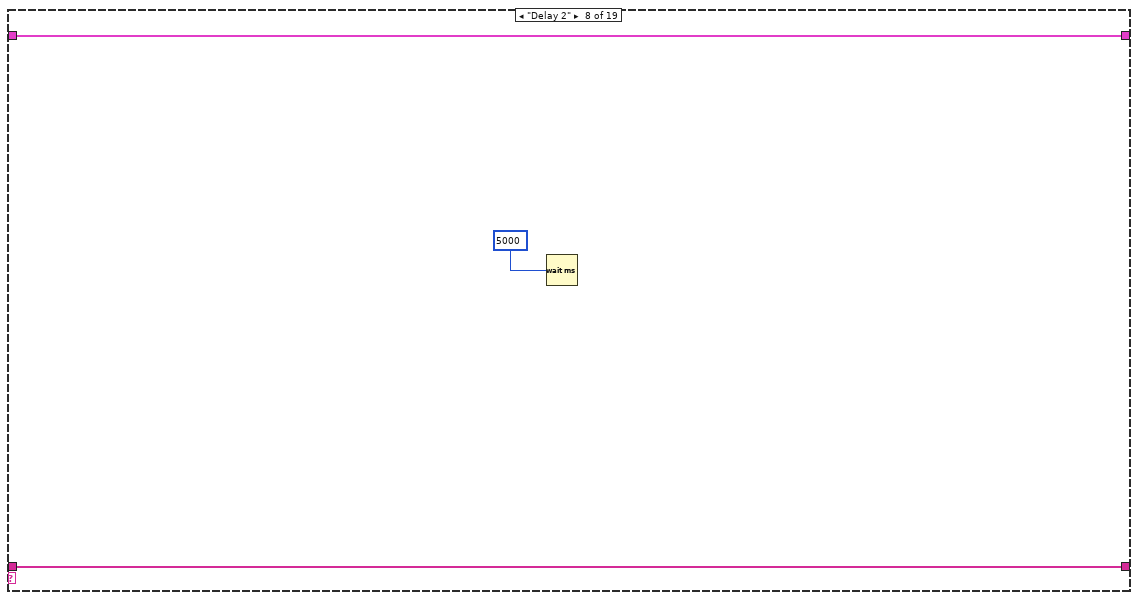
[diagram p11: hidden frame]
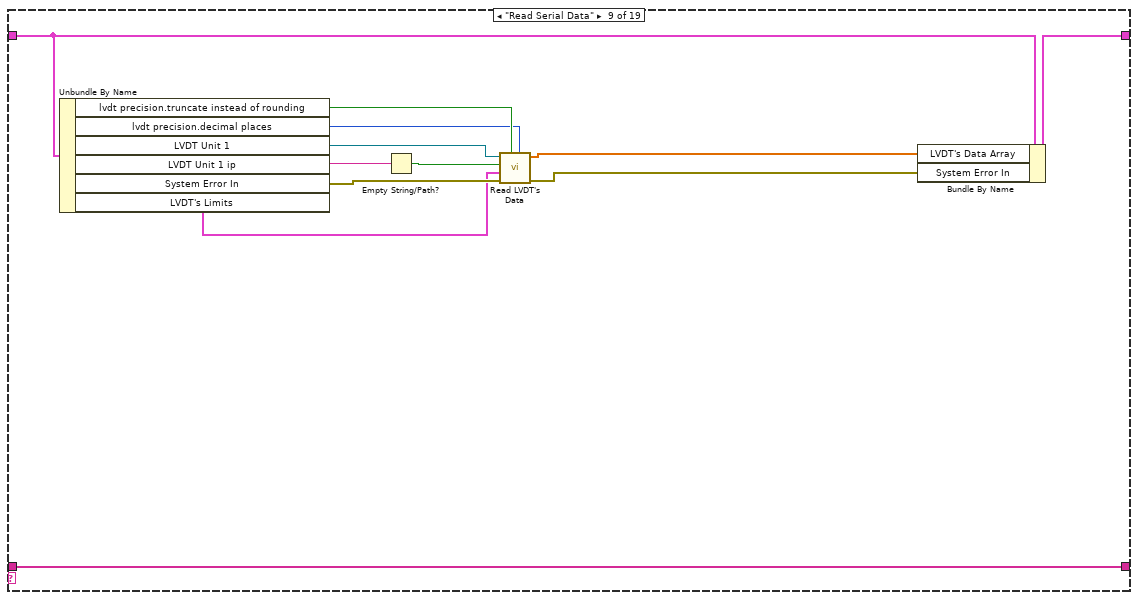
[diagram p12: hidden frame]
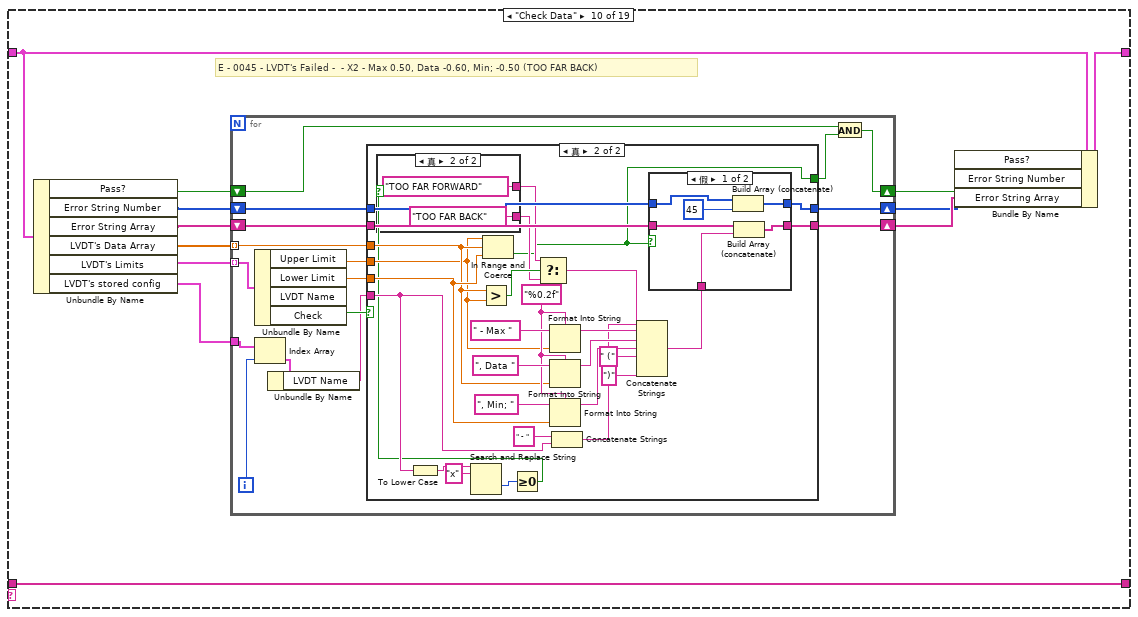
[diagram p13: hidden frame]
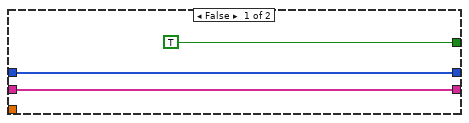
[diagram p14: hidden frame]
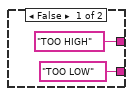
[diagram p15: hidden frame]
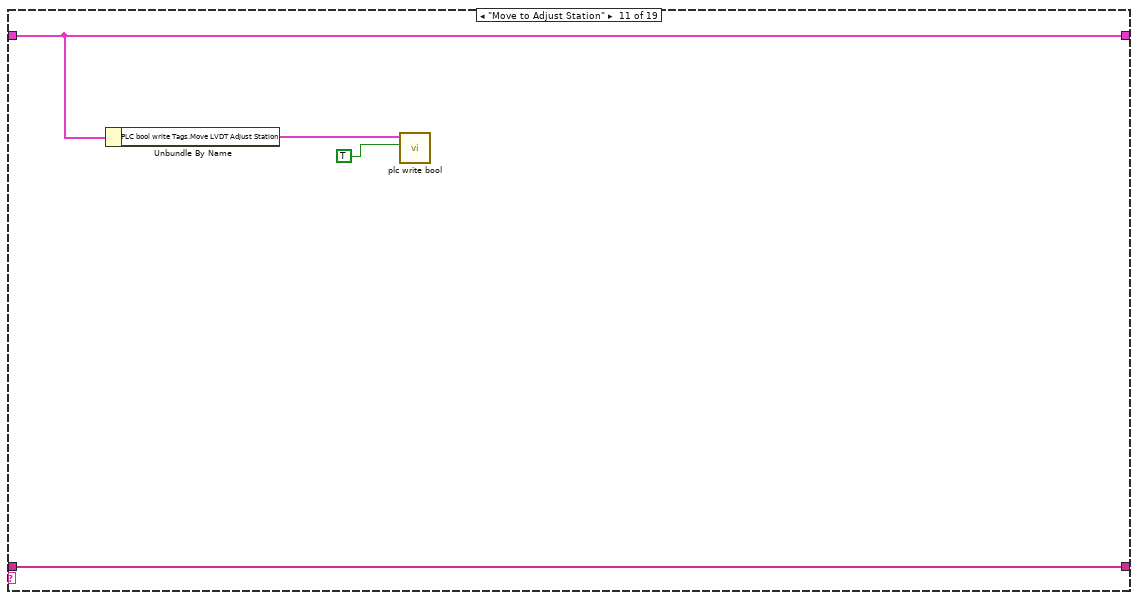
[diagram p17: hidden frame]
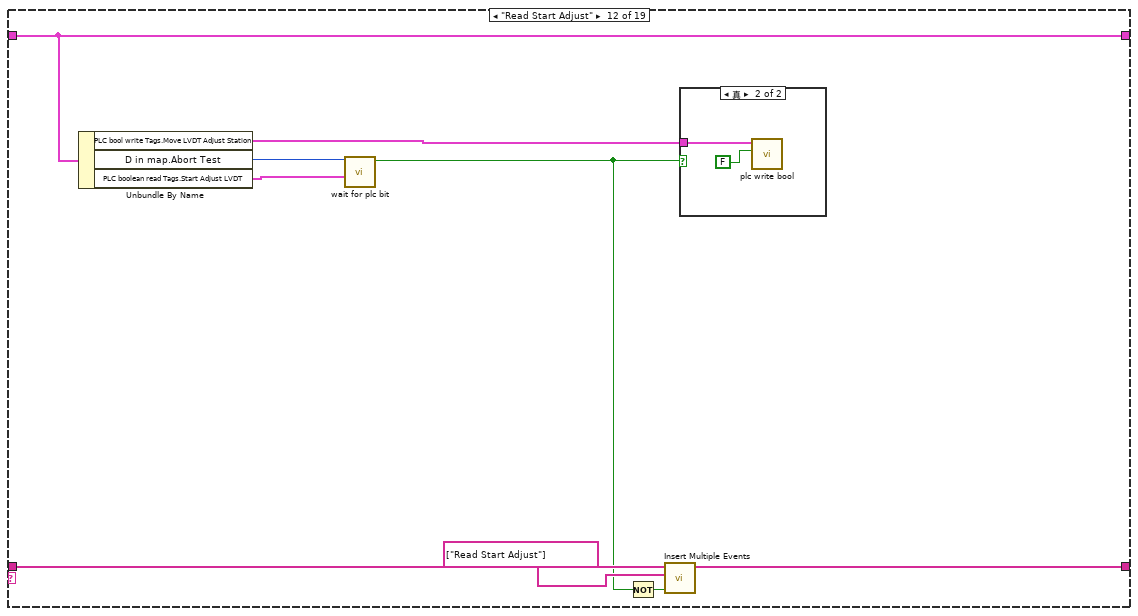
[diagram p18: hidden frame]
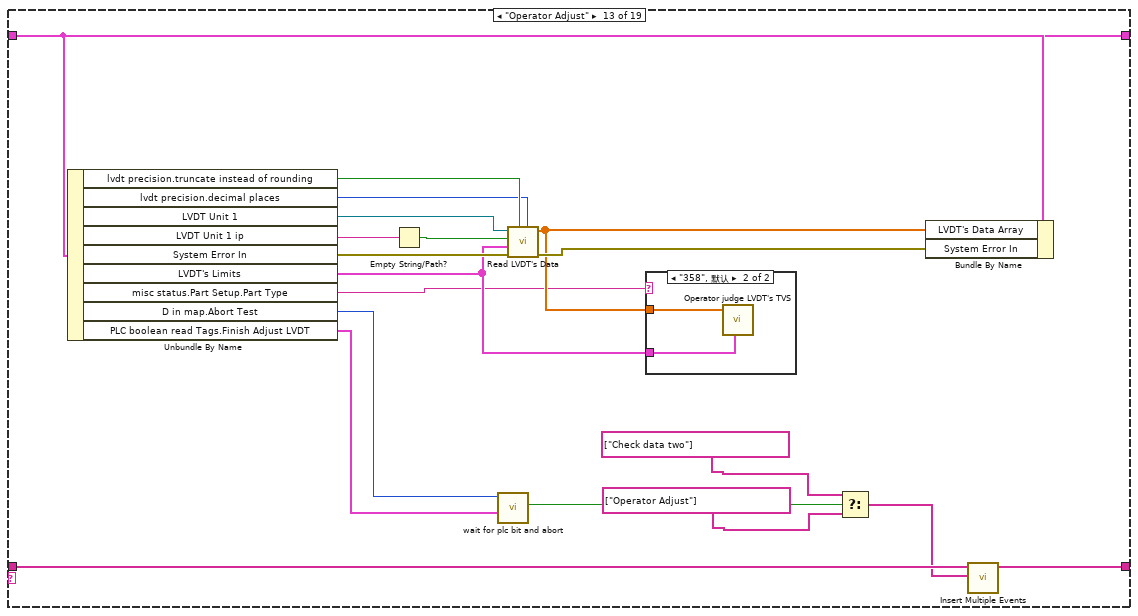
[diagram p20: hidden frame]
diagram:
  (unwired) string[] ["Extend LVDT's", "LVDT's Extended?", "Delay", "Read Serial Data", "Check Data", "Unextend LVDT's", "BJFA1", "Exit"] ("event queue out")
  w20 = T23[] []  # LVDT's Limits
  w18 = u16[] []  # Error String Number
  w19 = string[] []  # Error String Array
  w23 = TRUE  # Pass?
  w21 = sgl[] []  # LVDT's Data Array
  w22 = ""  # LVDT Data String
  # "Read Finish Adjust"
  # "Operator Adjust"
  # "Read Start Adjust"
  # "Move to Adjust Station"
  n1 = call "Config Info Get.vi"("Config Info"="input cluster") -> ("PLC Comms"=w3:T41)  [unwired: 7 in, 3 out]
  n2 = Unbundle By Name("input cluster") -> ("rs232 port map.LVDT Unit"=w10:refnum<visa-resource-name>, "Sequence State.Step Data String"=w16:string, "rs232 port map.LVDT Unit"=w14:refnum<visa-resource-name>, "D in map"=w15:T17, "LVDT Status.LVDT's stored config"=w12:T23[], "LVDT Status.lvdt precision"=w11:T24, "misc station config.use alt China TP2 LVDT Logic Seq"=w9:bool, "misc station config.use separate lvdt x and z extend tags"=w6:bool, "misc status"=w5:T47)
  n3 = Unbundle By Name(w3) -> ("PLC bool write Tags"=w1:T36, "PLC boolean read Tags"=w2:T42)
  n4 = Bundle(cluster=T40 {"Pass?"=FALSE, "LVDT Unit 1"="", "LVDT Data String"="", "LVDT's Data Array"=[], "LVDT's Limits"=[], "Error String Array"=[], "Error String Number"=[], "System Error In"={"status"=FALSE, "code"=0, "source"=""}, "Step Data String"="", "PLC bool write Tags"={"AT set glass wand lower"={"Tag Name"="", "Network Path"="", "use opc"=FALSE, "DataSocket Reference"={"CWDSLib._DCWDataSocket"=refnum, "CWDSLib._DCWData"=refnum, "OnDataUpdated"=0, "OnStatusUpdated"=0}}, "AT set sunshade wand lower"={"Tag Name"="", "Network Path"="", "use opc"=FALSE, "DataSocket Reference"={"CWDSLib._DCWDataSocket"=refnum, "CWDSLib._DCWData"=refnum, "OnDataUpdated"=0, "OnStatusUpdated"=0}}, "AT set wand home pos"={"Tag Name"="", "Network Path"="", "use opc"=FALSE, "DataSocket Reference"={"CWDSLib._DCWDataSocket"=refnum, "CWDSLib._DCWData"=refnum, "OnDataUpdated"=0, "OnStatusUpdated"=0}}, "Test Complete Pass"={"Tag Name"="", "Network Path"="", "use opc"=FALSE, "DataSocket Reference"={"CWDSLib._DCWDataSocket"=refnum, "CWDSLib._DCWData"=refnum, "OnDataUpdated"=0, "OnStatusUpdated"=0}}, "Test Complete Fail"={"Tag Name"="", "Network Path"="", "use opc"=FALSE, "DataSocket Reference"={"CWDSLib._DCWDataSocket"=refnum, "CWDSLib._DCWData"=refnum, "OnDataUpdated"=0, "OnStatusUpdated"=0}}, "Test Started"={"Tag Name"="", "Network Path"="", "use opc"=FALSE, "DataSocket Reference"={"CWDSLib._DCWDataSocket"=refnum, "CWDSLib._DCWData"=refnum, "OnDataUpdated"=0, "OnStatusUpdated"=0}}, "Retract LVDT's"={"Tag Name"="", "Network Path"="", "use opc"=FALSE, "DataSocket Reference"={"CWDSLib._DCWDataSocket"=refnum, "CWDSLib._DCWData"=refnum, "OnDataUpdated"=0, "OnStatusUpdated"=0}}, "Extend LVDT's"={"Tag Name"="", "Network Path"="", "use opc"=FALSE, "DataSocket Reference"={"CWDSLib._DCWDataSocket"=refnum, "CWDSLib._DCWData"=refnum, "OnDataUpdated"=0, "OnStatusUpdated"=0}}, "ss servo open"={"Tag Name"="", "Network Path"="", "use opc"=FALSE, "DataSocket Reference"={"CWDSLib._DCWDataSocket"=refnum, "CWDSLib._DCWData"=refnum, "OnDataUpdated"=0, "OnStatusUpdated"=0}}, "ss servo close"={"Tag Name"="", "Network Path"="", "use opc"=FALSE, "DataSocket Reference"={"CWDSLib._DCWDataSocket"=refnum, "CWDSLib._DCWData"=refnum, "OnDataUpdated"=0, "OnStatusUpdated"=0}}, "control slide start"={"Tag Name"="", "Network Path"="", "use opc"=FALSE, "DataSocket Reference"={"CWDSLib._DCWDataSocket"=refnum, "CWDSLib._DCWData"=refnum, "OnDataUpdated"=0, "OnStatusUpdated"=0}}, "control slide stop"={"Tag Name"="", "Network Path"="", "use opc"=FALSE, "DataSocket Reference"={"CWDSLib._DCWDataSocket"=refnum, "CWDSLib._DCWData"=refnum, "OnDataUpdated"=0, "OnStatusUpdated"=0}}, "AT VentPMACHome"={"Tag Name"="", "Network Path"="", "use opc"=FALSE, "DataSocket Reference"={"CWDSLib._DCWDataSocket"=refnum, "CWDSLib._DCWData"=refnum, "OnDataUpdated"=0, "OnStatusUpdated"=0}}, "AT VentPMACExtended"={"Tag Name"="", "Network Path"="", "use opc"=FALSE, "DataSocket Reference"={"CWDSLib._DCWDataSocket"=refnum, "CWDSLib._DCWData"=refnum, "OnDataUpdated"=0, "OnStatusUpdated"=0}}, "Good Frame Barcode"={"Tag Name"="", "Network Path"="", "use opc"=FALSE, "DataSocket Reference"={"CWDSLib._DCWDataSocket"=refnum, "CWDSLib._DCWData"=refnum, "OnDataUpdated"=0, "OnStatusUpdated"=0}}, "Bad Frame Barcode"={"Tag Name"="", "Network Path"="", "use opc"=FALSE, "DataSocket Reference"={"CWDSLib._DCWDataSocket"=refnum, "CWDSLib._DCWData"=refnum, "OnDataUpdated"=0, "OnStatusUpdated"=0}}, "Extend Z LVDTS"={"Tag Name"="", "Network Path"="", "use opc"=FALSE, "DataSocket Reference"={"CWDSLib._DCWDataSocket"=refnum, "CWDSLib._DCWData"=refnum, "OnDataUpdated"=0, "OnStatusUpdated"=0}}, "NVH SunRoof Moving"={"Tag Name"="", "Network Path"="", "use opc"=FALSE, "DataSocket Reference"={"CWDSLib._DCWDataSocket"=refnum, "CWDSLib._DCWData"=refnum, "OnDataUpdated"=0, "OnStatusUpdated"=0}}, "NVH SunRoof Stop"={"Tag Name"="", "Network Path"="", "use opc"=FALSE, "DataSocket Reference"={"CWDSLib._DCWDataSocket"=refnum, "CWDSLib._DCWData"=refnum, "OnDataUpdated"=0, "OnStatusUpdated"=0}}, "NVH Pass"={"Tag Name"="", "Network Path"="", "use opc"=FALSE, "DataSocket Reference"={"CWDSLib._DCWDataSocket"=refnum, "CWDSLib._DCWData"=refnum, "OnDataUpdated"=0, "OnStatusUpdated"=0}}, "NVH Fail"={"Tag Name"="", "Network Path"="", "use opc"=FALSE, "DataSocket Reference"={"CWDSLib._DCWDataSocket"=refnum, "CWDSLib._DCWData"=refnum, "OnDataUpdated"=0, "OnStatusUpdated"=0}}, "NVH Operator Express Glass Opened"={"Tag Name"="", "Network Path"="", "use opc"=FALSE, "DataSocket Reference"={"CWDSLib._DCWDataSocket"=refnum, "CWDSLib._DCWData"=refnum, "OnDataUpdated"=0, "OnStatusUpdated"=0}}, "NVH Operator Express Glass Closed"={"Tag Name"="", "Network Path"="", "use opc"=FALSE, "DataSocket Reference"={"CWDSLib._DCWDataSocket"=refnum, "CWDSLib._DCWData"=refnum, "OnDataUpdated"=0, "OnStatusUpdated"=0}}, "NVH Operator Express Rollo Opened01"={"Tag Name"="", "Network Path"="", "use opc"=FALSE, "DataSocket Reference"={"CWDSLib._DCWDataSocket"=refnum, "CWDSLib._DCWData"=refnum, "OnDataUpdated"=0, "OnStatusUpdated"=0}}, "NVH Operator Express Rollo Closed01"={"Tag Name"="", "Network Path"="", "use opc"=FALSE, "DataSocket Reference"={"CWDSLib._DCWDataSocket"=refnum, "CWDSLib._DCWData"=refnum, "OnDataUpdated"=0, "OnStatusUpdated"=0}}, "NVH Operator Express Rollo Opened02"={"Tag Name"="", "Network Path"="", "use opc"=FALSE, "DataSocket Reference"={"CWDSLib._DCWDataSocket"=refnum, "CWDSLib._DCWData"=refnum, "OnDataUpdated"=0, "OnStatusUpdated"=0}}, "NVH Operator Pass"={"Tag Name"="", "Network Path"="", "use opc"=FALSE, "DataSocket Reference"={"CWDSLib._DCWDataSocket"=refnum, "CWDSLib._DCWData"=refnum, "OnDataUpdated"=0, "OnStatusUpdated"=0}}, "NVH Operator Fail"={"Tag Name"="", "Network Path"="", "use opc"=FALSE, "DataSocket Reference"={"CWDSLib._DCWDataSocket"=refnum, "CWDSLib._DCWData"=refnum, "OnDataUpdated"=0, "OnStatusUpdated"=0}}, "NVH Operator Check"={"Tag Name"="", "Network Path"="", "use opc"=FALSE, "DataSocket Reference"={"CWDSLib._DCWDataSocket"=refnum, "CWDSLib._DCWData"=refnum, "OnDataUpdated"=0, "OnStatusUpdated"=0}}, "NVH Operator Vent Open Noise"={"Tag Name"="", "Network Path"="", "use opc"=FALSE, "DataSocket Reference"={"CWDSLib._DCWDataSocket"=refnum, "CWDSLib._DCWData"=refnum, "OnDataUpdated"=0, "OnStatusUpdated"=0}}, "NVH Operator Vent Close Noise"={"Tag Name"="", "Network Path"="", "use opc"=FALSE, "DataSocket Reference"={"CWDSLib._DCWDataSocket"=refnum, "CWDSLib._DCWData"=refnum, "OnDataUpdated"=0, "OnStatusUpdated"=0}}, "NVH Operator Sunshade Open Noise"={"Tag Name"="", "Network Path"="", "use opc"=FALSE, "DataSocket Reference"={"CWDSLib._DCWDataSocket"=refnum, "CWDSLib._DCWData"=refnum, "OnDataUpdated"=0, "OnStatusUpdated"=0}}, "NVH Operator Sunshade Close Noise"={"Tag Name"="", "Network Path"="", "use opc"=FALSE, "DataSocket Reference"={"CWDSLib._DCWDataSocket"=refnum, "CWDSLib._DCWData"=refnum, "OnDataUpdated"=0, "OnStatusUpdated"=0}}, "NVH Operator Glass Open Noise"={"Tag Name"="", "Network Path"="", "use opc"=FALSE, "DataSocket Reference"={"CWDSLib._DCWDataSocket"=refnum, "CWDSLib._DCWData"=refnum, "OnDataUpdated"=0, "OnStatusUpdated"=0}}, "NVH Operator Glass Close Noise"={"Tag Name"="", "Network Path"="", "use opc"=FALSE, "DataSocket Reference"={"CWDSLib._DCWDataSocket"=refnum, "CWDSLib._DCWData"=refnum, "OnDataUpdated"=0, "OnStatusUpdated"=0}}, "NVH Operator Finish"={"Tag Name"="", "Network Path"="", "use opc"=FALSE, "DataSocket Reference"={"CWDSLib._DCWDataSocket"=refnum, "CWDSLib._DCWData"=refnum, "OnDataUpdated"=0, "OnStatusUpdated"=0}}, "AT set sunshade 02 wand up"={"Tag Name"="", "Network Path"="", "use opc"=FALSE, "DataSocket Reference"={"CWDSLib._DCWDataSocket"=refnum, "CWDSLib._DCWData"=refnum, "OnDataUpdated"=0, "OnStatusUpdated"=0}}, "AT set wand 02 home pos"={"Tag Name"="", "Network Path"="", "use opc"=FALSE, "DataSocket Reference"={"CWDSLib._DCWDataSocket"=refnum, "CWDSLib._DCWData"=refnum, "OnDataUpdated"=0, "OnStatusUpdated"=0}}, "Barcode01 OK"={"Tag Name"="", "Network Path"="", "use opc"=FALSE, "DataSocket Reference"={"CWDSLib._DCWDataSocket"=refnum, "CWDSLib._DCWData"=refnum, "OnDataUpdated"=0, "OnStatusUpdated"=0}}, "Barcode02 OK"={"Tag Name"="", "Network Path"="", "use opc"=FALSE, "DataSocket Reference"={"CWDSLib._DCWDataSocket"=refnum, "CWDSLib._DCWData"=refnum, "OnDataUpdated"=0, "OnStatusUpdated"=0}}, "AT set to Vent ATS Test Pos"={"Tag Name"="", "Network Path"="", "use opc"=FALSE, "DataSocket Reference"={"CWDSLib._DCWDataSocket"=refnum, "CWDSLib._DCWData"=refnum, "OnDataUpdated"=0, "OnStatusUpdated"=0}}, "AT set to Vent ATS Home Pos"={"Tag Name"="", "Network Path"="", "use opc"=FALSE, "DataSocket Reference"={"CWDSLib._DCWDataSocket"=refnum, "CWDSLib._DCWData"=refnum, "OnDataUpdated"=0, "OnStatusUpdated"=0}}, "Move LVDT Adjust Station"={"Tag Name"="", "Network Path"="", "use opc"=FALSE, "DataSocket Reference"={"CWDSLib._DCWDataSocket"=refnum, "CWDSLib._DCWData"=refnum, "OnDataUpdated"=0, "OnStatusUpdated"=0}}}, "PLC boolean read Tags"={"AT glass position"={"Tag Name"="", "Network Path"="", "use opc"=FALSE, "DataSocket Reference"={"CWDSLib._DCWDataSocket"=refnum, "CWDSLib._DCWData"=refnum, "OnDataUpdated"=0, "OnStatusUpdated"=0}}, "AT shade position"={"Tag Name"="", "Network Path"="", "use opc"=FALSE, "DataSocket Reference"={"CWDSLib._DCWDataSocket"=refnum, "CWDSLib._DCWData"=refnum, "OnDataUpdated"=0, "OnStatusUpdated"=0}}, "AT in glass wand lower pos"={"Tag Name"="", "Network Path"="", "use opc"=FALSE, "DataSocket Reference"={"CWDSLib._DCWDataSocket"=refnum, "CWDSLib._DCWData"=refnum, "OnDataUpdated"=0, "OnStatusUpdated"=0}}, "AT in sunshad wand lower pos"={"Tag Name"="", "Network Path"="", "use opc"=FALSE, "DataSocket Reference"={"CWDSLib._DCWDataSocket"=refnum, "CWDSLib._DCWData"=refnum, "OnDataUpdated"=0, "OnStatusUpdated"=0}}, "AT in wand home pos"={"Tag Name"="", "Network Path"="", "use opc"=FALSE, "DataSocket Reference"={"CWDSLib._DCWDataSocket"=refnum, "CWDSLib._DCWData"=refnum, "OnDataUpdated"=0, "OnStatusUpdated"=0}}, "LVDT's Extended"={"Tag Name"="", "Network Path"="", "use opc"=FALSE, "DataSocket Reference"={"CWDSLib._DCWDataSocket"=refnum, "CWDSLib._DCWData"=refnum, "OnDataUpdated"=0, "OnStatusUpdated"=0}}, "motor foam present LH"={"Tag Name"="", "Network Path"="", "use opc"=FALSE, "DataSocket Reference"={"CWDSLib._DCWDataSocket"=refnum, "CWDSLib._DCWData"=refnum, "OnDataUpdated"=0, "OnStatusUpdated"=0}}, "motor foam present RH"={"Tag Name"="", "Network Path"="", "use opc"=FALSE, "DataSocket Reference"={"CWDSLib._DCWDataSocket"=refnum, "CWDSLib._DCWData"=refnum, "OnDataUpdated"=0, "OnStatusUpdated"=0}}, "audit gap hider present LH"={"Tag Name"="", "Network Path"="", "use opc"=FALSE, "DataSocket Reference"={"CWDSLib._DCWDataSocket"=refnum, "CWDSLib._DCWData"=refnum, "OnDataUpdated"=0, "OnStatusUpdated"=0}}, "audit gap hider present RH"={"Tag Name"="", "Network Path"="", "use opc"=FALSE, "DataSocket Reference"={"CWDSLib._DCWDataSocket"=refnum, "CWDSLib._DCWData"=refnum, "OnDataUpdated"=0, "OnStatusUpdated"=0}}, "FB light block present"={"Tag Name"="", "Network Path"="", "use opc"=FALSE, "DataSocket Reference"={"CWDSLib._DCWDataSocket"=refnum, "CWDSLib._DCWData"=refnum, "OnDataUpdated"=0, "OnStatusUpdated"=0}}, "bolt check 1"={"Tag Name"="", "Network Path"="", "use opc"=FALSE, "DataSocket Reference"={"CWDSLib._DCWDataSocket"=refnum, "CWDSLib._DCWData"=refnum, "OnDataUpdated"=0, "OnStatusUpdated"=0}}, "bolt check 2"={"Tag Name"="", "Network Path"="", "use opc"=FALSE, "DataSocket Reference"={"CWDSLib._DCWDataSocket"=refnum, "CWDSLib._DCWData"=refnum, "OnDataUpdated"=0, "OnStatusUpdated"=0}}, "bolt check 3"={"Tag Name"="", "Network Path"="", "use opc"=FALSE, "DataSocket Reference"={"CWDSLib._DCWDataSocket"=refnum, "CWDSLib._DCWData"=refnum, "OnDataUpdated"=0, "OnStatusUpdated"=0}}, "bolt check 4"={"Tag Name"="", "Network Path"="", "use opc"=FALSE, "DataSocket Reference"={"CWDSLib._DCWDataSocket"=refnum, "CWDSLib._DCWData"=refnum, "OnDataUpdated"=0, "OnStatusUpdated"=0}}, "bolt check 5"={"Tag Name"="", "Network Path"="", "use opc"=FALSE, "DataSocket Reference"={"CWDSLib._DCWDataSocket"=refnum, "CWDSLib._DCWData"=refnum, "OnDataUpdated"=0, "OnStatusUpdated"=0}}, "bolt check 6"={"Tag Name"="", "Network Path"="", "use opc"=FALSE, "DataSocket Reference"={"CWDSLib._DCWDataSocket"=refnum, "CWDSLib._DCWData"=refnum, "OnDataUpdated"=0, "OnStatusUpdated"=0}}, "bolt check 7"={"Tag Name"="", "Network Path"="", "use opc"=FALSE, "DataSocket Reference"={"CWDSLib._DCWDataSocket"=refnum, "CWDSLib._DCWData"=refnum, "OnDataUpdated"=0, "OnStatusUpdated"=0}}, "bolt check 8"={"Tag Name"="", "Network Path"="", "use opc"=FALSE, "DataSocket Reference"={"CWDSLib._DCWDataSocket"=refnum, "CWDSLib._DCWData"=refnum, "OnDataUpdated"=0, "OnStatusUpdated"=0}}, "bolt check 9"={"Tag Name"="", "Network Path"="", "use opc"=FALSE, "DataSocket Reference"={"CWDSLib._DCWDataSocket"=refnum, "CWDSLib._DCWData"=refnum, "OnDataUpdated"=0, "OnStatusUpdated"=0}}, "bolt check 10"={"Tag Name"="", "Network Path"="", "use opc"=FALSE, "DataSocket Reference"={"CWDSLib._DCWDataSocket"=refnum, "CWDSLib._DCWData"=refnum, "OnDataUpdated"=0, "OnStatusUpdated"=0}}, "bolt check 11"={"Tag Name"="", "Network Path"="", "use opc"=FALSE, "DataSocket Reference"={"CWDSLib._DCWDataSocket"=refnum, "CWDSLib._DCWData"=refnum, "OnDataUpdated"=0, "OnStatusUpdated"=0}}, "bolt check 12"={"Tag Name"="", "Network Path"="", "use opc"=FALSE, "DataSocket Reference"={"CWDSLib._DCWDataSocket"=refnum, "CWDSLib._DCWData"=refnum, "OnDataUpdated"=0, "OnStatusUpdated"=0}}, "bolt check 13"={"Tag Name"="", "Network Path"="", "use opc"=FALSE, "DataSocket Reference"={"CWDSLib._DCWDataSocket"=refnum, "CWDSLib._DCWData"=refnum, "OnDataUpdated"=0, "OnStatusUpdated"=0}}, "bolt check 14"={"Tag Name"="", "Network Path"="", "use opc"=FALSE, "DataSocket Reference"={"CWDSLib._DCWDataSocket"=refnum, "CWDSLib._DCWData"=refnum, "OnDataUpdated"=0, "OnStatusUpdated"=0}}, "bolt check 15"={"Tag Name"="", "Network Path"="", "use opc"=FALSE, "DataSocket Reference"={"CWDSLib._DCWDataSocket"=refnum, "CWDSLib._DCWData"=refnum, "OnDataUpdated"=0, "OnStatusUpdated"=0}}, "bolt check 16"={"Tag Name"="", "Network Path"="", "use opc"=FALSE, "DataSocket Reference"={"CWDSLib._DCWDataSocket"=refnum, "CWDSLib._DCWData"=refnum, "OnDataUpdated"=0, "OnStatusUpdated"=0}}, "bolt check 17"={"Tag Name"="", "Network Path"="", "use opc"=FALSE, "DataSocket Reference"={"CWDSLib._DCWDataSocket"=refnum, "CWDSLib._DCWData"=refnum, "OnDataUpdated"=0, "OnStatusUpdated"=0}}, "bolt check 18"={"Tag Name"="", "Network Path"="", "use opc"=FALSE, "DataSocket Reference"={"CWDSLib._DCWDataSocket"=refnum, "CWDSLib._DCWData"=refnum, "OnDataUpdated"=0, "OnStatusUpdated"=0}}, "bolt check 19"={"Tag Name"="", "Network Path"="", "use opc"=FALSE, "DataSocket Reference"={"CWDSLib._DCWDataSocket"=refnum, "CWDSLib._DCWData"=refnum, "OnDataUpdated"=0, "OnStatusUpdated"=0}}, "bolt check 20"={"Tag Name"="", "Network Path"="", "use opc"=FALSE, "DataSocket Reference"={"CWDSLib._DCWDataSocket"=refnum, "CWDSLib._DCWData"=refnum, "OnDataUpdated"=0, "OnStatusUpdated"=0}}, "bolt check 21"={"Tag Name"="", "Network Path"="", "use opc"=FALSE, "DataSocket Reference"={"CWDSLib._DCWDataSocket"=refnum, "CWDSLib._DCWData"=refnum, "OnDataUpdated"=0, "OnStatusUpdated"=0}}, "start"={"Tag Name"="", "Network Path"="", "use opc"=FALSE, "DataSocket Reference"={"CWDSLib._DCWDataSocket"=refnum, "CWDSLib._DCWData"=refnum, "OnDataUpdated"=0, "OnStatusUpdated"=0}}, "abort"={"Tag Name"="", "Network Path"="", "use opc"=FALSE, "DataSocket Reference"={"CWDSLib._DCWDataSocket"=refnum, "CWDSLib._DCWData"=refnum, "OnDataUpdated"=0, "OnStatusUpdated"=0}}, "LVDT's Retracted"={"Tag Name"="", "Network Path"="", "use opc"=FALSE, "DataSocket Reference"={"CWDSLib._DCWDataSocket"=refnum, "CWDSLib._DCWData"=refnum, "OnDataUpdated"=0, "OnStatusUpdated"=0}}, "manual barcode print"={"Tag Name"="", "Network Path"="", "use opc"=FALSE, "DataSocket Reference"={"CWDSLib._DCWDataSocket"=refnum, "CWDSLib._DCWData"=refnum, "OnDataUpdated"=0, "OnStatusUpdated"=0}}, "ss servo at open"={"Tag Name"="", "Network Path"="", "use opc"=FALSE, "DataSocket Reference"={"CWDSLib._DCWDataSocket"=refnum, "CWDSLib._DCWData"=refnum, "OnDataUpdated"=0, "OnStatusUpdated"=0}}, "ss servo at close"={"Tag Name"="", "Network Path"="", "use opc"=FALSE, "DataSocket Reference"={"CWDSLib._DCWDataSocket"=refnum, "CWDSLib._DCWData"=refnum, "OnDataUpdated"=0, "OnStatusUpdated"=0}}, "ss servo opening"={"Tag Name"="", "Network Path"="", "use opc"=FALSE, "DataSocket Reference"={"CWDSLib._DCWDataSocket"=refnum, "CWDSLib._DCWData"=refnum, "OnDataUpdated"=0, "OnStatusUpdated"=0}}, "ss servo closing"={"Tag Name"="", "Network Path"="", "use opc"=FALSE, "DataSocket Reference"={"CWDSLib._DCWDataSocket"=refnum, "CWDSLib._DCWData"=refnum, "OnDataUpdated"=0, "OnStatusUpdated"=0}}, "control slide at home"={"Tag Name"="", "Network Path"="", "use opc"=FALSE, "DataSocket Reference"={"CWDSLib._DCWDataSocket"=refnum, "CWDSLib._DCWData"=refnum, "OnDataUpdated"=0, "OnStatusUpdated"=0}}, "control slide left good"={"Tag Name"="", "Network Path"="", "use opc"=FALSE, "DataSocket Reference"={"CWDSLib._DCWDataSocket"=refnum, "CWDSLib._DCWData"=refnum, "OnDataUpdated"=0, "OnStatusUpdated"=0}}, "control slide left over stroke"={"Tag Name"="", "Network Path"="", "use opc"=FALSE, "DataSocket Reference"={"CWDSLib._DCWDataSocket"=refnum, "CWDSLib._DCWData"=refnum, "OnDataUpdated"=0, "OnStatusUpdated"=0}}, "control slide right good"={"Tag Name"="", "Network Path"="", "use opc"=FALSE, "DataSocket Reference"={"CWDSLib._DCWDataSocket"=refnum, "CWDSLib._DCWData"=refnum, "OnDataUpdated"=0, "OnStatusUpdated"=0}}, "control slide right over stroke"={"Tag Name"="", "Network Path"="", "use opc"=FALSE, "DataSocket Reference"={"CWDSLib._DCWDataSocket"=refnum, "CWDSLib._DCWData"=refnum, "OnDataUpdated"=0, "OnStatusUpdated"=0}}, "wind deflector high speed pos"={"Tag Name"="", "Network Path"="", "use opc"=FALSE, "DataSocket Reference"={"CWDSLib._DCWDataSocket"=refnum, "CWDSLib._DCWData"=refnum, "OnDataUpdated"=0, "OnStatusUpdated"=0}}, "wind deflector low speed pos"={"Tag Name"="", "Network Path"="", "use opc"=FALSE, "DataSocket Reference"={"CWDSLib._DCWDataSocket"=refnum, "CWDSLib._DCWData"=refnum, "OnDataUpdated"=0, "OnStatusUpdated"=0}}, "AT VentPMACatHome"={"Tag Name"="", "Network Path"="", "use opc"=FALSE, "DataSocket Reference"={"CWDSLib._DCWDataSocket"=refnum, "CWDSLib._DCWData"=refnum, "OnDataUpdated"=0, "OnStatusUpdated"=0}}, "AT VentPMACisExtend"={"Tag Name"="", "Network Path"="", "use opc"=FALSE, "DataSocket Reference"={"CWDSLib._DCWDataSocket"=refnum, "CWDSLib._DCWData"=refnum, "OnDataUpdated"=0, "OnStatusUpdated"=0}}, "SS Barcode Scanner Bypassed"={"Tag Name"="", "Network Path"="", "use opc"=FALSE, "DataSocket Reference"={"CWDSLib._DCWDataSocket"=refnum, "CWDSLib._DCWData"=refnum, "OnDataUpdated"=0, "OnStatusUpdated"=0}}, "Check Frame Barcode"={"Tag Name"="", "Network Path"="", "use opc"=FALSE, "DataSocket Reference"={"CWDSLib._DCWDataSocket"=refnum, "CWDSLib._DCWData"=refnum, "OnDataUpdated"=0, "OnStatusUpdated"=0}}, "iGPS Pass 0"={"Tag Name"="", "Network Path"="", "use opc"=FALSE, "DataSocket Reference"={"CWDSLib._DCWDataSocket"=refnum, "CWDSLib._DCWData"=refnum, "OnDataUpdated"=0, "OnStatusUpdated"=0}}, "iGPS Pass 1"={"Tag Name"="", "Network Path"="", "use opc"=FALSE, "DataSocket Reference"={"CWDSLib._DCWDataSocket"=refnum, "CWDSLib._DCWData"=refnum, "OnDataUpdated"=0, "OnStatusUpdated"=0}}, "iGPS Pass 2"={"Tag Name"="", "Network Path"="", "use opc"=FALSE, "DataSocket Reference"={"CWDSLib._DCWDataSocket"=refnum, "CWDSLib._DCWData"=refnum, "OnDataUpdated"=0, "OnStatusUpdated"=0}}, "iGPS Pass 3"={"Tag Name"="", "Network Path"="", "use opc"=FALSE, "DataSocket Reference"={"CWDSLib._DCWDataSocket"=refnum, "CWDSLib._DCWData"=refnum, "OnDataUpdated"=0, "OnStatusUpdated"=0}}, "iGPS Pass 4"={"Tag Name"="", "Network Path"="", "use opc"=FALSE, "DataSocket Reference"={"CWDSLib._DCWDataSocket"=refnum, "CWDSLib._DCWData"=refnum, "OnDataUpdated"=0, "OnStatusUpdated"=0}}, "iGPS Pass 5"={"Tag Name"="", "Network Path"="", "use opc"=FALSE, "DataSocket Reference"={"CWDSLib._DCWDataSocket"=refnum, "CWDSLib._DCWData"=refnum, "OnDataUpdated"=0, "OnStatusUpdated"=0}}, "iGPS Pass 6"={"Tag Name"="", "Network Path"="", "use opc"=FALSE, "DataSocket Reference"={"CWDSLib._DCWDataSocket"=refnum, "CWDSLib._DCWData"=refnum, "OnDataUpdated"=0, "OnStatusUpdated"=0}}, "iGPS Pass 7"={"Tag Name"="", "Network Path"="", "use opc"=FALSE, "DataSocket Reference"={"CWDSLib._DCWDataSocket"=refnum, "CWDSLib._DCWData"=refnum, "OnDataUpdated"=0, "OnStatusUpdated"=0}}, "iGPS Pass 8"={"Tag Name"="", "Network Path"="", "use opc"=FALSE, "DataSocket Reference"={"CWDSLib._DCWDataSocket"=refnum, "CWDSLib._DCWData"=refnum, "OnDataUpdated"=0, "OnStatusUpdated"=0}}, "iGPS Pass 9"={"Tag Name"="", "Network Path"="", "use opc"=FALSE, "DataSocket Reference"={"CWDSLib._DCWDataSocket"=refnum, "CWDSLib._DCWData"=refnum, "OnDataUpdated"=0, "OnStatusUpdated"=0}}, "Z LVDTs Extended"={"Tag Name"="", "Network Path"="", "use opc"=FALSE, "DataSocket Reference"={"CWDSLib._DCWDataSocket"=refnum, "CWDSLib._DCWData"=refnum, "OnDataUpdated"=0, "OnStatusUpdated"=0}}, "NVH Operator Pass"={"Tag Name"="", "Network Path"="", "use opc"=FALSE, "DataSocket Reference"={"CWDSLib._DCWDataSocket"=refnum, "CWDSLib._DCWData"=refnum, "OnDataUpdated"=0, "OnStatusUpdated"=0}}, "NVH Operator Fail"={"Tag Name"="", "Network Path"="", "use opc"=FALSE, "DataSocket Reference"={"CWDSLib._DCWDataSocket"=refnum, "CWDSLib._DCWData"=refnum, "OnDataUpdated"=0, "OnStatusUpdated"=0}}, "NVH Operator Express Glass Open"={"Tag Name"="", "Network Path"="", "use opc"=FALSE, "DataSocket Reference"={"CWDSLib._DCWDataSocket"=refnum, "CWDSLib._DCWData"=refnum, "OnDataUpdated"=0, "OnStatusUpdated"=0}}, "NVH Operator Express Glass Close"={"Tag Name"="", "Network Path"="", "use opc"=FALSE, "DataSocket Reference"={"CWDSLib._DCWDataSocket"=refnum, "CWDSLib._DCWData"=refnum, "OnDataUpdated"=0, "OnStatusUpdated"=0}}, "NVH Operator Express Rollo Open01"={"Tag Name"="", "Network Path"="", "use opc"=FALSE, "DataSocket Reference"={"CWDSLib._DCWDataSocket"=refnum, "CWDSLib._DCWData"=refnum, "OnDataUpdated"=0, "OnStatusUpdated"=0}}, "NVH Operator Express Rollo Close01"={"Tag Name"="", "Network Path"="", "use opc"=FALSE, "DataSocket Reference"={"CWDSLib._DCWDataSocket"=refnum, "CWDSLib._DCWData"=refnum, "OnDataUpdated"=0, "OnStatusUpdated"=0}}, "NVH Operator Express Rollo Open02"={"Tag Name"="", "Network Path"="", "use opc"=FALSE, "DataSocket Reference"={"CWDSLib._DCWDataSocket"=refnum, "CWDSLib._DCWData"=refnum, "OnDataUpdated"=0, "OnStatusUpdated"=0}}, "NVH Operator Express Rollo Close02"={"Tag Name"="", "Network Path"="", "use opc"=FALSE, "DataSocket Reference"={"CWDSLib._DCWDataSocket"=refnum, "CWDSLib._DCWData"=refnum, "OnDataUpdated"=0, "OnStatusUpdated"=0}}, "NVH Operator Vent Open Noise"={"Tag Name"="", "Network Path"="", "use opc"=FALSE, "DataSocket Reference"={"CWDSLib._DCWDataSocket"=refnum, "CWDSLib._DCWData"=refnum, "OnDataUpdated"=0, "OnStatusUpdated"=0}}, "NVH Operator Vent Close Noise"={"Tag Name"="", "Network Path"="", "use opc"=FALSE, "DataSocket Reference"={"CWDSLib._DCWDataSocket"=refnum, "CWDSLib._DCWData"=refnum, "OnDataUpdated"=0, "OnStatusUpdated"=0}}, "NVH Operator Sunshade Open Noise"={"Tag Name"="", "Network Path"="", "use opc"=FALSE, "DataSocket Reference"={"CWDSLib._DCWDataSocket"=refnum, "CWDSLib._DCWData"=refnum, "OnDataUpdated"=0, "OnStatusUpdated"=0}}, "NVH Operator Sunshade Close Noise"={"Tag Name"="", "Network Path"="", "use opc"=FALSE, "DataSocket Reference"={"CWDSLib._DCWDataSocket"=refnum, "CWDSLib._DCWData"=refnum, "OnDataUpdated"=0, "OnStatusUpdated"=0}}, "NVH Operator Glass Open Noise"={"Tag Name"="", "Network Path"="", "use opc"=FALSE, "DataSocket Reference"={"CWDSLib._DCWDataSocket"=refnum, "CWDSLib._DCWData"=refnum, "OnDataUpdated"=0, "OnStatusUpdated"=0}}, "NVH Operator Glass Close Noise"={"Tag Name"="", "Network Path"="", "use opc"=FALSE, "DataSocket Reference"={"CWDSLib._DCWDataSocket"=refnum, "CWDSLib._DCWData"=refnum, "OnDataUpdated"=0, "OnStatusUpdated"=0}}, "NVH Operator Finish"={"Tag Name"="", "Network Path"="", "use opc"=FALSE, "DataSocket Reference"={"CWDSLib._DCWDataSocket"=refnum, "CWDSLib._DCWData"=refnum, "OnDataUpdated"=0, "OnStatusUpdated"=0}}, "NVH Operator Check"={"Tag Name"="", "Network Path"="", "use opc"=FALSE, "DataSocket Reference"={"CWDSLib._DCWDataSocket"=refnum, "CWDSLib._DCWData"=refnum, "OnDataUpdated"=0, "OnStatusUpdated"=0}}, "AT shade 02 position"={"Tag Name"="", "Network Path"="", "use opc"=FALSE, "DataSocket Reference"={"CWDSLib._DCWDataSocket"=refnum, "CWDSLib._DCWData"=refnum, "OnDataUpdated"=0, "OnStatusUpdated"=0}}, "AT in sunshad 02 wand up pos"={"Tag Name"="", "Network Path"="", "use opc"=FALSE, "DataSocket Reference"={"CWDSLib._DCWDataSocket"=refnum, "CWDSLib._DCWData"=refnum, "OnDataUpdated"=0, "OnStatusUpdated"=0}}, "AT in wand 02 home pos"={"Tag Name"="", "Network Path"="", "use opc"=FALSE, "DataSocket Reference"={"CWDSLib._DCWDataSocket"=refnum, "CWDSLib._DCWData"=refnum, "OnDataUpdated"=0, "OnStatusUpdated"=0}}, "windproof position"={"Tag Name"="", "Network Path"="", "use opc"=FALSE, "DataSocket Reference"={"CWDSLib._DCWDataSocket"=refnum, "CWDSLib._DCWData"=refnum, "OnDataUpdated"=0, "OnStatusUpdated"=0}}, "NVH Operator Express Glass vent Open"={"Tag Name"="", "Network Path"="", "use opc"=FALSE, "DataSocket Reference"={"CWDSLib._DCWDataSocket"=refnum, "CWDSLib._DCWData"=refnum, "OnDataUpdated"=0, "OnStatusUpdated"=0}}, "NVH Operator Express Glass Vent Close"={"Tag Name"="", "Network Path"="", "use opc"=FALSE, "DataSocket Reference"={"CWDSLib._DCWDataSocket"=refnum, "CWDSLib._DCWData"=refnum, "OnDataUpdated"=0, "OnStatusUpdated"=0}}, "NVH Operator Re-do"={"Tag Name"="", "Network Path"="", "use opc"=FALSE, "DataSocket Reference"={"CWDSLib._DCWDataSocket"=refnum, "CWDSLib._DCWData"=refnum, "OnDataUpdated"=0, "OnStatusUpdated"=0}}, "AT at vent ATS test pos"={"Tag Name"="", "Network Path"="", "use opc"=FALSE, "DataSocket Reference"={"CWDSLib._DCWDataSocket"=refnum, "CWDSLib._DCWData"=refnum, "OnDataUpdated"=0, "OnStatusUpdated"=0}}, "AT at vent ATS Home pos"={"Tag Name"="", "Network Path"="", "use opc"=FALSE, "DataSocket Reference"={"CWDSLib._DCWDataSocket"=refnum, "CWDSLib._DCWData"=refnum, "OnDataUpdated"=0, "OnStatusUpdated"=0}}, "Start Adjust LVDT"={"Tag Name"="", "Network Path"="", "use opc"=FALSE, "DataSocket Reference"={"CWDSLib._DCWDataSocket"=refnum, "CWDSLib._DCWData"=refnum, "OnDataUpdated"=0, "OnStatusUpdated"=0}}, "Finish Adjust LVDT"={"Tag Name"="", "Network Path"="", "use opc"=FALSE, "DataSocket Reference"={"CWDSLib._DCWDataSocket"=refnum, "CWDSLib._DCWData"=refnum, "OnDataUpdated"=0, "OnStatusUpdated"=0}}}, "D in map"={"Abort Test"=enum."Dev2/port0/line0", "Start Test"=enum."Dev2/port0/line0"}, "LVDT's stored config"=[], "lvdt precision"={"truncate instead of rounding"=FALSE, "decimal places"=0}, "LVDT Unit 1 ip"="", "use alt China TP2 LVDT Logic Seq"=FALSE, "check lvdt x?"=FALSE, "separate z extend"=FALSE, "misc status"={"delay start time (ticks)"=0, "In Vehicle Mode?"=FALSE, "Diag Mode?"=FALSE, "Serial Port Configured?"=FALSE, "PS Voltage"=0.0, "Diag Serial Port"="", "Part Setup"={"Communication Type"=enum."None", "Send Messages to"=enum."Glass", "RAP Signal"=enum."High", "Motor Type"=enum."Smart Motor", "NVH Part Number"=0, "Turn Off Timer"=0, "Part Type"=""}, "Part History Number"="", "Plant Number"=0, "AP Data Type"=enum."91/61", "Real Rollo?"=FALSE}}, "Pass?"=w23, "LVDT Unit 1"=w14, "LVDT Data String"=w22, "LVDT's Data Array"=w21, "LVDT's Limits"=w20, "Error String Array"=w19, "Error String Number"=w18, "System Error In"="System Error In", "Step Data String"=w16, "PLC bool write Tags"=w1, "PLC boolean read Tags"=w2, "D in map"=w15, "LVDT's stored config"=w12, "lvdt precision"=w11, "LVDT Unit 1 ip"=w10, "use alt China TP2 LVDT Logic Seq"=w9, "check lvdt x?"="check lvdt x?", "separate z extend"=w6, "misc status"=w5) -> (w13:T40)
  n5 = while {
    shift-right: [w33] -> _
    shift-left: string[] ["Init"] ("event queue out") -> [w29]
    shift-right: [w32] -> _
    shift-left: w13 -> [w26]
    tunnel: "input cluster" -> [w25]
    stop <- w30 continue-if-true
    n6 = call "EOL next state.vi"("Main State Cluster"=w25, "event queue in"=w29) -> ("Condition (Exit:F)"=w30:bool, "next event"=w27:string, "event queue out"=w28:string[])  [unwired: 5 in, 2 out]
    n7 = Wait (ms)(milliseconds to wait=u32 10) -> ()  [unwired: 1 out]
    n8 = case shown="\"LVDT's Unextended?\"" w27 {
      tunnel: w28 -> [_ _ w53 w62 w87 w101 w118 w121 w135 w137 w208 w216 w233 w249 w330 w363 w378 w393 w421]
      tunnel: [string[] ["Exit"] ("event queue out") w39 w53 w61 w87 w100 w118 w121 w135 w137 w208 w217 w232 w249 w330 w362 w378 w392 w421] -> w33
      tunnel: w26 -> [w34 w49 w52 w60 w86 w99 w119 w122 w134 w143 w209 w215 w235 w248 w325 w349 w377 w385 w420]
      tunnel: [w34 w45 w52 w59 w86 w98 w119 w122 w133 w142 w209 w215 w234 w250 w325 w358 w377 w384 w420] -> w32
      frame "Error", Default {
      }
      frame "Init" {
        n9 = Unbundle By Name(w49) -> ("LVDT's Limits"=w48:T23[], "Step Data String"=w47:string, "System Error In"=w46:errorcluster, "use alt China TP2 LVDT Logic Seq"=w42:bool, "check lvdt x?"=w41:bool)  [unwired: 2 out]
        n10 = Unflatten From String(type=w48, binary string=w47, error in (no error)=w46) -> (value=w44:T23[], error out=w37:errorcluster)  [unwired: 2 in, 1 out]
        n11 = Select(t=string[] ["Extend LVDT's", "LVDT's Extended?", "Delay", "Read Serial Data", "Check Data", "Unextend LVDT's", "LVDT's Unextended?", "Reset LVDT's Slide Down", "Exit"] ("event queue out"), s=w42, f=string[] ["Extend LVDT's", "LVDT's Extended?", "Delay", "Read Serial Data", "Check Data", "Unextend LVDT's", "LVDT's Unextended?", "Exit"] ("event queue out")) -> (s? t:f=w38:string[])
        n12 = Bundle By Name(cluster=w49, "LVDT's Limits"=w44, "System Error In"=w37) -> (w45:T40)
        n13 = Select(t=string[] ["Set LVDT's Slide Down", "Check LVDT's Slide Down", "Extend LVDT's", "LVDT's Extended?", "Delay", "Read Serial Data", "Check Data", "Unextend LVDT's", "LVDT's Unextended?", "Reset LVDT's Slide Down", "Check Reset LVDT's Slide Down", "Exit"] ("event queue out"), s=w41, f=w38) -> (s? t:f=w39:string[])
      }
      frame "Set LVDT's Slide Down" {
        n14 = Unbundle By Name(w52) -> ("PLC bool write Tags.Retract LVDT's"=w50:T37)
        n15 = call "plc write bool.vi"("value"=TRUE, "addr,tag"=w50) -> ()  [unwired: 9 in, 1 out]
      }
      frame "Check LVDT's Slide Down" {
        (unwired) 45000 ("timeout (ms)")
        n16 = Unbundle By Name(w60) -> ("Pass?"=w64:bool, "Error String Array"=w66:string[], "Error String Number"=w58:u16[], "D in map.Abort Test"=w55:T18, "PLC boolean read Tags.LVDT's Retracted"=w54:T37)
        n17 = call "wait for plc bit.vi"("tag"=w54, "Abort Test"=w55) -> ("final values"=w56:bool)  [unwired: 8 in, 1 out]
        n18 = case shown="假" w56 {
          tunnel: w66 -> [w70 w78]
          tunnel: [w71 w78] -> w65
          tunnel: w64 -> [_ w77]
          tunnel: [FALSE ("Pass?") w77] -> w63
          tunnel: w58 -> [w74 w76]
          tunnel: [w72 w76] -> w57
          frame False {
            n19 = Build Array (concatenate)(w70, "-") -> (w71:string[])
            n20 = Build Array (concatenate)(w74, u16 43 ("read tags")) -> (w72:u16[])
          }
          frame True {
          }
        }
        n21 = Not(x=w56) -> (.not. x?=w68:bool)
        n22 = Bundle By Name(cluster=w60, "Pass?"=w63, "Error String Array"=w65, "Error String Number"=w57) -> (w59:T40)
        n23 = call "Insert Multiple Events.vi"("Insert all? (T)"=w68, "Events to Insert"=string[] ["Exit"], "Event queue in"=w62) -> ("Event queue out"=w61:string[])  [unwired: 4 in]
      }
      frame "Extend LVDT's" {
        n24 = Unbundle By Name(w86) -> ("PLC bool write Tags.Extend Z LVDTS"=w81:T37, "separate z extend"=w84:bool, "check lvdt x?"=w82:bool, "PLC bool write Tags.Extend LVDT's"=w80:T37)
        n25 = Compound Arithmetic op=AND(w84, invert w82) -> (w83:bool)
        n26 = Select(t=w81, s=w83, f=w80) -> (s? t:f=w79:T37)
        n27 = call "plc write bool.vi"("value"=TRUE, "addr,tag"=w79) -> ()  [unwired: 9 in, 1 out]
      }
      frame "LVDT's Extended?" {
        n28 = Unbundle By Name(w99) -> ("Pass?"=w103:bool, "Error String Array"=w105:string[], "Error String Number"=w97:u16[], "D in map.Abort Test"=w95:T18, "PLC boolean read Tags.LVDT's Extended"=w90:T37, "PLC boolean read Tags.Z LVDTs Extended"=w91:T37, "separate z extend"=w92:bool, "check lvdt x?"=w93:bool)
        n29 = Compound Arithmetic op=AND(w92, invert w93) -> (w94:bool)
        n30 = Select(t=w91, s=w94, f=w90) -> (s? t:f=w89:T37)
        n31 = call "wait for plc bit.vi"("tag"=w89, "Abort Test"=w95) -> ("final values"=w88:bool)  [unwired: 8 in, 1 out]
        n32 = case shown="假" w88 {
          tunnel: w105 -> [w109 w117]
          tunnel: [w110 w117] -> w104
          tunnel: w103 -> [_ w116]
          tunnel: [FALSE ("Pass?") w116] -> w102
          tunnel: w97 -> [w113 w115]
          tunnel: [w111 w115] -> w96
          frame False {
            n33 = Build Array (concatenate)(w109, "-") -> (w110:string[])
            n34 = Build Array (concatenate)(w113, u16 43 ("read tags")) -> (w111:u16[])
          }
          frame True {
          }
        }
        n35 = Not(x=w88) -> (.not. x?=w107:bool)
        n36 = Bundle By Name(cluster=w99, "Pass?"=w102, "Error String Array"=w104, "Error String Number"=w96) -> (w98:T40)
        n37 = call "Insert Multiple Events.vi"("Insert all? (T)"=w107, "Events to Insert"=string[] ["Exit"], "Event queue in"=w101) -> ("Event queue out"=w100:string[])  [unwired: 4 in]
      }
      frame "Delay" {
        n38 = Wait (ms)(milliseconds to wait=u32 1000) -> ()  [unwired: 1 out]
      }
      frame "Delay 2" {
        n39 = Wait (ms)(milliseconds to wait=u32 5000) -> ()  [unwired: 1 out]
      }
      frame "Read Serial Data" {
        n40 = Unbundle By Name(w134) -> ("lvdt precision.truncate instead of rounding"=w129:bool, "lvdt precision.decimal places"=w128:u8, "LVDT Unit 1"=w131:refnum<visa-resource-name>, "LVDT Unit 1 ip"=w132:string, "System Error In"=w125:errorcluster, "LVDT's Limits"=w124:T23[])
        n41 = Empty String/Path?(string/path=w132) -> (empty?=w130:bool)
        n42 = call "Read LVDT's Data.vi"("Desired Decimal Points"=w128, "truncate instead of round"=w129, "error in"=w125, "LVDT's Limits"=w124, "rs232?"=w130, "LVDT's Com Port"=w131) -> ("error out"=w126:errorcluster, "Array"=w127:sgl[])  [unwired: 4 in]
        n43 = Bundle By Name(cluster=w134, "LVDT's Data Array"=w127, "System Error In"=w126) -> (w133:T40)
      }
      frame "Check Data" {
        # "E - 0045 - LVDT's Failed -  - X2 - Max 0.50, Data -0.60, Min; -0.50 (TOO FAR BACK)"
        n44 = Unbundle By Name(w143) -> ("Pass?"=w144:bool, "Error String Number"=w140:u16[], "Error String Array"=w145:string[], "LVDT's Data Array"=w147:sgl[], "LVDT's Limits"=w146:T23[], "LVDT's stored config"=w138:T23[])
        n45 = for {
          tunnel: w147 -> [w163] mode=indexing
          tunnel: w146 -> [w160] mode=indexing
          shift-right: [w156] -> w141
          shift-left: w145 -> [w155]
          shift-right: [w161] -> w136
          shift-left: w144 -> [w162]
          shift-right: [w154] -> w139
          shift-left: w140 -> [w153]
          tunnel: w138 -> [w151]
          i -> [w150]
          n46 = Unbundle By Name(w160) -> ("Upper Limit"=w159:dbl, "Lower Limit"=w158:dbl, "Check"=w152:bool)  [unwired: 1 out]
          n47 = Index Array(array=w151, index=w150) -> (element=w149:T23)
          n48 = Unbundle By Name(w149) -> ("LVDT Name"=w148:string)
          n49 = case shown="真" w152 {
            tunnel: w163 -> [_ w178]
            tunnel: w159 -> [_ w177]
            tunnel: w158 -> [_ w186]
            tunnel: w148 -> [_ w172]
            tunnel: [TRUE w167] -> w157
            tunnel: [w164 w184] -> w156
            tunnel: w155 -> [w164 w183]
            tunnel: [w165 w182] -> w154
            tunnel: w153 -> [w165 w181]
            frame False {
            }
            frame True {
              w189 = "%0.2f" ("format string")
              n50 = To Lower Case(string=w172) -> (all lower case string=w171:string)
              n51 = Search and Replace String(input string=w171, search string="x") -> (offset past replacement=w169:i32)  [unwired: 6 in, 3 out]
              n52 = Greater?(x=w178, y=w177) -> (0:w176:bool)
              n53 = In Range and Coerce(upper limit=w177, x=w178, lower limit=w186) -> (In Range?=w167:bool)  [unwired: 1 out]
              n54 = Greater Or Equal To 0?(x=w169) -> (x >= 0?=w168:bool)
              n55 = case shown="真" w168 {
                tunnel: ["TOO HIGH" ("initial string") "TOO FAR FORWARD" ("initial string")] -> w175
                tunnel: ["TOO LOW" ("initial string") "TOO FAR BACK" ("initial string")] -> w174
                frame False {
                }
                frame True {
                }
              }
              n56 = Select(t=w175, s=w176, f=w174) -> (s? t:f=w173:string)
              n57 = Format Into String(format string=w189, initial string=" - Max ", w177) -> (resulting string=w192:string)  [unwired: 1 in, 1 out]
              n58 = Format Into String(format string=w189, initial string=", Data ", w178) -> (resulting string=w191:string)  [unwired: 1 in, 1 out]
              n59 = Format Into String(format string=w189, initial string=", Min; ", w186) -> (resulting string=w190:string)  [unwired: 1 in, 1 out]
              n60 = Concatenate Strings(" - " ("initial string"), w172) -> (w187:string)
              n61 = Concatenate Strings(w187, w192, w191, w190, " (" ("string"), w173, ")" ("string")) -> (w185:string)
              n62 = case shown="假" w167 {
                tunnel: w185 -> [w205 _]
                tunnel: [w204 w207] -> w184
                tunnel: w183 -> [w203 w207]
                tunnel: [w201 w206] -> w182
                tunnel: w181 -> [w200 w206]
                frame False {
                  n63 = Build Array (concatenate)(w200, u8 45 ("Error No.")) -> (w201:u16[])
                  n64 = Build Array (concatenate)(w203, w205) -> (w204:string[])
                }
                frame True {
                }
              }
            }
          }
          n65 = And(x=w162, y=w157) -> (x .and. y?=w161:bool)
        }
        n66 = Bundle By Name(cluster=w143, "Pass?"=w136, "Error String Number"=w139, "Error String Array"=w141) -> (w142:T40)
      }
      frame "Move to Adjust Station" {
        n67 = Unbundle By Name(w209) -> ("PLC bool write Tags.Move LVDT Adjust Station"=w210:T37)
        n68 = call "plc write bool.vi"("value"=TRUE, "addr,tag"=w210) -> ()  [unwired: 9 in, 1 out]
      }
      frame "Read Start Adjust" {
        n69 = Unbundle By Name(w215) -> ("PLC bool write Tags.Move LVDT Adjust Station"=w212:T37, "D in map.Abort Test"=w219:T18, "PLC boolean read Tags.Start Adjust LVDT"=w220:T37)
        n70 = call "wait for plc bit.vi"("tag"=w220, "Abort Test"=w219) -> ("final values"=w213:bool)  [unwired: 8 in, 1 out]
        n71 = Not(x=w213) -> (.not. x?=w214:bool)
        n72 = call "Insert Multiple Events.vi"("Insert all? (T)"=w214, "Events to Insert"=string[] ["Read Start Adjust"], "Event queue in"=w216) -> ("Event queue out"=w217:string[])  [unwired: 4 in]
        n73 = case shown="真" w213 {
          tunnel: w212 -> [_ w221]
          frame False {
          }
          frame True {
            n74 = call "plc write bool.vi"("value"=FALSE, "addr,tag"=w221) -> ()  [unwired: 9 in, 1 out]
          }
        }
      }
      frame "Operator Adjust" {
        n75 = Unbundle By Name(w235) -> ("lvdt precision.truncate instead of rounding"=w239:bool, "lvdt precision.decimal places"=w238:u8, "LVDT Unit 1"=w241:refnum<visa-resource-name>, "LVDT Unit 1 ip"=w242:string, "System Error In"=w236:errorcluster, "LVDT's Limits"=w228:T23[], "misc status.Part Setup.Part Type"=w226:string, "D in map.Abort Test"=w225:T18, "PLC boolean read Tags.Finish Adjust LVDT"=w224:T37)
        n76 = Empty String/Path?(string/path=w242) -> (empty?=w240:bool)
        n77 = call "wait for plc bit and abort.vi"("tag"=w224, "Abort Test"=w225) -> ("final values"=w223:bool)  [unwired: 8 in, 1 out]
        n78 = call "Read LVDT's Data.vi"("Desired Decimal Points"=w238, "truncate instead of round"=w239, "error in"=w236, "LVDT's Limits"=w228, "rs232?"=w240, "LVDT's Com Port"=w241) -> ("error out"=w237:errorcluster, "Array"=w227:sgl[])  [unwired: 4 in]
        n79 = case shown="\"358\", 默认" w226 {
          tunnel: w228 -> [w243 w245]
          tunnel: w227 -> [w244 w246]
          frame "CX11" {
            n80 = call "Operator judge LVDT's TP.vi"("LVDT's Limits"=w243, "LVDT's Array"=w244) -> ()  [unwired: 10 in]
          }
          frame "358", Default {
            n81 = call "Operator judge LVDT's TVS.vi"("LVDT's Limits"=w245, "LVDT's Array"=w246) -> ()  [unwired: 10 in]
          }
        }
        n82 = Select(t=string[] ["Check data two"] ("Events to Insert"), s=w223, f=string[] ["Operator Adjust"] ("Events to Insert")) -> (s? t:f=w229:string[])
        n83 = Bundle By Name(cluster=w235, "LVDT's Data Array"=w227, "System Error In"=w237) -> (w234:T40)
        n84 = call "Insert Multiple Events.vi"("Events to Insert"=w229, "Event queue in"=w233) -> ("Event queue out"=w232:string[])  [unwired: 5 in]
      }
      frame "Check data two" {
        # "E - 0045 - LVDT's Failed -  - X2 - Max 0.50, Data -0.60, Min; -0.50 (TOO FAR BACK)"
        n85 = Unbundle By Name(w248) -> ("Error String Number"=w254:u16[], "Error String Array"=w256:string[], "LVDT's Data Array"=w258:sgl[], "LVDT's Limits"=w257:T23[], "LVDT's stored config"=w252:T23[])
        n86 = for {
          tunnel: w258 -> [w274] mode=indexing
          tunnel: w257 -> [w271] mode=indexing
          shift-right: [w267] -> w255
          shift-left: w256 -> [w266]
          shift-right: [w272] -> w251
          shift-left: TRUE -> [w273]
          shift-right: [w265] -> w253
          shift-left: w254 -> [w264]
          tunnel: w252 -> [w262]
          i -> [w261]
          n87 = Unbundle By Name(w271) -> ("Upper Limit"=w270:dbl, "Lower Limit"=w269:dbl, "Check"=w263:bool)  [unwired: 1 out]
          n88 = Index Array(array=w262, index=w261) -> (element=w260:T23)
          n89 = Unbundle By Name(w260) -> ("LVDT Name"=w259:string)
          n90 = case shown="真" w263 {
            tunnel: w274 -> [_ w288]
            tunnel: w270 -> [_ w287]
            tunnel: w269 -> [_ w297]
            tunnel: w259 -> [_ w282]
            tunnel: [TRUE w296] -> w268
            tunnel: [w275 w294] -> w267
            tunnel: w266 -> [w275 w293]
            tunnel: [w276 w292] -> w265
            tunnel: w264 -> [w276 w291]
            frame False {
            }
            frame True {
              w300 = "%0.2f" ("format string")
              n91 = To Lower Case(string=w282) -> (all lower case string=w281:string)
              n92 = Search and Replace String(input string=w281, search string="x") -> (offset past replacement=w279:i32)  [unwired: 6 in, 3 out]
              n93 = Greater?(x=w288, y=w287) -> (0:w286:bool)
              n94 = In Range and Coerce(upper limit=w287, x=w288, lower limit=w297) -> (In Range?=w296:bool)  [unwired: 1 out]
              n95 = Greater Or Equal To 0?(x=w279) -> (x >= 0?=w278:bool)
              n96 = case shown="真" w278 {
                tunnel: ["TOO HIGH" ("initial string") "TOO FAR FORWARD" ("initial string")] -> w285
                tunnel: ["TOO LOW" ("initial string") "TOO FAR BACK" ("initial string")] -> w284
                frame False {
                }
                frame True {
                }
              }
              n97 = Select(t=w285, s=w286, f=w284) -> (s? t:f=w283:string)
              n98 = Format Into String(format string=w300, initial string=" - Max ", w287) -> (resulting string=w303:string)  [unwired: 1 in, 1 out]
              n99 = Format Into String(format string=w300, initial string=", Data ", w288) -> (resulting string=w302:string)  [unwired: 1 in, 1 out]
              n100 = Format Into String(format string=w300, initial string=", Min; ", w297) -> (resulting string=w301:string)  [unwired: 1 in, 1 out]
              n101 = Concatenate Strings(" - " ("initial string"), w282) -> (w298:string)
              n102 = Concatenate Strings(w298, w303, w302, w301, " (" ("string"), w283, ")" ("string")) -> (w295:string)
              n103 = case shown="假" w296 {
                tunnel: w295 -> [w316 _]
                tunnel: [w315 w318] -> w294
                tunnel: w293 -> [w314 w318]
                tunnel: [w312 w317] -> w292
                tunnel: w291 -> [w311 w317]
                frame False {
                  n104 = Build Array (concatenate)(w311, u8 45 ("Error No.")) -> (w312:u16[])
                  n105 = Build Array (concatenate)(w314, w316) -> (w315:string[])
                }
                frame True {
                }
              }
            }
          }
          n106 = And(x=w273, y=w268) -> (x .and. y?=w272:bool)
        }
        n107 = Bundle By Name(cluster=w248, "Pass?"=w251, "Error String Number"=w253, "Error String Array"=w255) -> (w250:T40)
      }
      frame "Unextend LVDT's" {
        n108 = Unbundle By Name(w325) -> ("PLC bool write Tags.Retract LVDT's"=w326:T37, "PLC bool write Tags.Extend LVDT's"=w320:T37, "use alt China TP2 LVDT Logic Seq"=w327:bool, "PLC bool write Tags.Extend Z LVDTS"=w321:T37, "separate z extend"=w323:bool, "check lvdt x?"=w322:bool)
        n109 = Compound Arithmetic op=AND(w323, invert w322) -> (w324:bool)
        n110 = Select(t=w321, s=w324, f=w320) -> (s? t:f=w319:T37)
        n111 = flat-sequence {
          tunnel: w319 -> [w333]
          tunnel: [w332] -> w329
          tunnel: w326 -> [w332]
          tunnel: [w331] -> w328
          tunnel: w327 -> [w331]
          tunnel: w329 -> [w336]
          tunnel: w328 -> [w335]
          frame #0 {
            n112 = call "plc write bool.vi"("value"=FALSE, "addr,tag"=w333) -> ()  [unwired: 9 in, 1 out]
          }
          frame #1 {
            n113 = case shown="真" w335 {
              tunnel: w336 -> [_ w337]
              frame False {
              }
              frame True {
                n114 = call "plc write bool.vi"("value"=TRUE, "addr,tag"=w337) -> ()  [unwired: 9 in, 1 out]
              }
            }
          }
        }
      }
      frame "LVDT's Unextended?" {
        (unwired) 10000 ("timeout (ms)")
        n115 = Unbundle By Name(w349) -> ("Pass?"=w348:bool, "Error String Array"=w347:string[], "Error String Number"=w346:u16[], "D in map.Abort Test"=w350:T18, "PLC boolean read Tags.LVDT's Extended"=w340:T37, "PLC boolean read Tags.LVDT's Retracted"=w351:T37, "use alt China TP2 LVDT Logic Seq"=w356:bool, "PLC boolean read Tags.Z LVDTs Extended"=w341:T37, "separate z extend"=w342:bool, "check lvdt x?"=w343:bool)
        n116 = Compound Arithmetic op=AND(w342, invert w343) -> (w344:bool)
        n117 = Select(t=FALSE, s=w356, f=TRUE ("inverse")) -> (s? t:f=w354:bool)
        n118 = Select(t=w341, s=w344, f=w340) -> (s? t:f=w339:T37)
        n119 = Select(t=w351, s=w356, f=w339) -> (s? t:f=w352:T37)
        n120 = call "wait for plc bit.vi"("inverse"=w354, "tag"=w352, "Abort Test"=w350) -> ("final values"=w345:bool)  [unwired: 7 in, 1 out]
        n121 = Not(x=w345) -> (.not. x?=w357:bool)
        n122 = case shown="假" w345 {
          tunnel: w347 -> [w366 w374]
          tunnel: [w367 w374] -> w361
          tunnel: w348 -> [_ w373]
          tunnel: [FALSE ("Pass?") w373] -> w360
          tunnel: w346 -> [w370 w372]
          tunnel: [w368 w372] -> w359
          frame False {
            n123 = Build Array (concatenate)(w366, "-") -> (w367:string[])
            n124 = Build Array (concatenate)(w370, u16 44 ("read tags")) -> (w368:u16[])
          }
          frame True {
          }
        }
        n125 = Bundle By Name(cluster=w349, "Pass?"=w360, "Error String Array"=w361, "Error String Number"=w359) -> (w358:T40)
        n126 = call "Insert Multiple Events.vi"("Insert all? (T)"=w357, "Events to Insert"=string[] ["Exit"], "Event queue in"=w363) -> ("Event queue out"=w362:string[])  [unwired: 4 in]
      }
      frame "Reset LVDT's Slide Down" {
        n127 = Unbundle By Name(w377) -> ("PLC bool write Tags.Retract LVDT's"=w375:T37)
        n128 = call "plc write bool.vi"("value"=FALSE, "addr,tag"=w375) -> ()  [unwired: 9 in, 1 out]
      }
      frame "Check Reset LVDT's Slide Down" {
        (unwired) 45000 ("timeout (ms)")
        n129 = Unbundle By Name(w385) -> ("Pass?"=w389:bool, "Error String Array"=w391:string[], "Error String Number"=w387:u16[], "PLC boolean read Tags.LVDT's Retracted"=w382:T37, "D in map.Abort Test"=w383:T18)
        n130 = call "wait for plc bit.vi"("inverse"=TRUE, "tag"=w382, "Abort Test"=w383) -> ("final values"=w380:bool)  [unwired: 7 in, 1 out]
        n131 = case shown="假" w380 {
          tunnel: w391 -> [w396 w404]
          tunnel: [w397 w404] -> w390
          tunnel: w389 -> [_ w403]
          tunnel: [FALSE ("Pass?") w403] -> w388
          tunnel: w387 -> [w400 w402]
          tunnel: [w398 w402] -> w386
          frame False {
            n132 = Build Array (concatenate)(w396, "-") -> (w397:string[])
            n133 = Build Array (concatenate)(w400, u16 44 ("read tags")) -> (w398:u16[])
          }
          frame True {
          }
        }
        n134 = Not(x=w380) -> (.not. x?=w379:bool)
        n135 = Bundle By Name(cluster=w385, "Pass?"=w388, "Error String Array"=w390, "Error String Number"=w386) -> (w384:T40)
        n136 = call "Insert Multiple Events.vi"("Insert all? (T)"=w379, "Events to Insert"=string[] ["Exit"], "Event queue in"=w393) -> ("Event queue out"=w392:string[])  [unwired: 4 in]
      }
      frame "Exit" {
        n137 = Unbundle By Name(w420) -> ("LVDT Unit 1 ip"=w408:string, "Pass?"=→"Pass?":bool, "System Error In"=w406:errorcluster, "Error String Array"=→"Error String Array":string[], "Error String Number"=→"Error String Number":u16[], "LVDT's Data Array"=w419:sgl[], "LVDT's Limits"=w418:T23[], "LVDT's stored config"=w410:T23[])
        n138 = for {
          tunnel: w419 -> [w426] mode=indexing
          tunnel: w418 -> [w438] mode=indexing
          shift-right: [w432] -> w414
          shift-left: "Database LVDT's Data In" -> [w437]
          tunnel: w410 -> [w430]
          tunnel: [w425] -> w409 mode=indexing if=w424
          i -> [w429]
          n139 = Index Array(array=w430, index=w429) -> (element=w431:T23)
          n140 = Unbundle By Name(w438) -> ("Lower Limit"=w435:dbl, "Upper Limit"=w436:dbl, "Check"=w424:bool)
          n141 = Unbundle By Name(w431) -> ("LVDT Name"=w427:string)
          n142 = Multiply(x=w429, y=3) -> (x*y=w433:i32)
          n143 = case shown="真" w424 {
            tunnel: w437 -> [w439 w447]
            tunnel: w426 -> [_ w446]
            tunnel: w436 -> [_ w445]
            tunnel: w435 -> [_ w444]
            tunnel: w433 -> [_ w443]
            tunnel: [w439 w440] -> w432
            frame False {
            }
            frame True {
              n144 = Increment(x=w443) -> (x+1=w442:i32)
              n145 = Increment(x=w442) -> (x+1=w441:i32)
              n146 = Replace Array Subset(array=w447, new element #1=w446, index #1=w443, new element #2=w444, index #2=w442, new element #3=w445, index #3=w441) -> (w440:sgl[])
            }
          }
          n147 = Bundle By Name(cluster=T1 {"lvdt name"="", "value"=0.0} ("lvdt name-val"), "lvdt name"=w427, "value"=w426) -> (w425:T1)
        }
        "Database LVDT's Data Out" <- w414
        n148 = Empty String/Path?(string/path=w408) -> (empty?=w407:bool)
        n149 = case shown="假" w407 {
          tunnel: w406 -> [w422 w423]
          tunnel: [w422 w423] -> w405
          frame False {
            # "***if we need to \nexplicitly close connection"
          }
          frame True {
          }
        }
        "System Error Out" <- w405
        n150 = Build Array (concatenate)("lvdt display in", w409) -> (→"lvdt display out":T1[])
      }
    }
  }
